vi "PJ1_ui-commu_1_test_4_Harmonics.vi"() -> ()   [LabVIEW 2024]
uses:
  contron/Control 7.ctl
  contron/Control 6.ctl
  contron/Control 5.ctl
  contron/Control 8.ctl
  contol_vr 23/66.ctl
  contol_vr 23/6.ctl
  <vilib>/express/express analysis/Spectral/Block/exnSpectralBlock spectral measurements PSD poly.vi
  <vilib>/express/express analysis/Spectral/XNode/ExpressSpectralMeasurementsBlockNode.xnode
  <vilib>/express/express analysis/Spectral/Block/exnSpectralBlock spectral measurements PSD DDT.vi
panel:
  out "PSD 24-1":dbl
  out "B 24-1":dbl
  in  "Aj 24-1":dbl
  out "B 33-1":dbl
  out "N 33-1":dbl
  in  "Aj 33-1":dbl
  out "B 33-1":dbl
  out "PSD 33-1":dbl
  out "B 33":dbl
  out "N 33":dbl
  in  "Aj 33":dbl
  out "B 33":dbl
  out "PSD 33":dbl
  out "B 33+1":dbl
  out "N 33+1":dbl
  in  "Aj 33+1":dbl
  out "B 33+1":dbl
  out "PSD 33+1":dbl
  out "B24-1":dbl
  out "N 24-1":dbl
  out "B 24":dbl
  out "N 24":dbl
  in  "Aj 24":dbl
  out "B  24":dbl
  out "PSD 24":dbl
  out "B 24+1":dbl
  out "N 24+1":dbl
  in  "Aj 24+1":dbl
  out "B 24+1":dbl
  out "PSD 24+1":dbl
  out "B21-1":dbl
  out "N21-1":dbl
  in  "Aj 21-1":dbl
  out "B  21-1":dbl
  out "PSD 21-1":dbl
  out "B21":dbl
  out "N21":dbl
  in  "Aj 21":dbl
  out "B  21":dbl
  out "PSD 21":dbl
  out "B21+1":dbl
  out "N21+1":dbl
  in  "Aj 21+1":dbl
  out "B  21+1":dbl
  out "PSD 21+1":dbl
  out "B18+1":dbl
  out "N18+1":dbl
  in  "Aj 18+1":dbl
  out "B  18+1":dbl
  out "PSD 18+1":dbl
  out "B18":dbl
  out "N18":dbl
  in  "Aj 18":dbl
  out "B  18":dbl
  out "PSD 18":dbl
  out "B18-1":dbl
  out "N18-1":dbl
  in  "Aj 18-1":dbl
  out "B  18-1":dbl
  out "PSD 18-1":dbl
  out "appended array 2":dbl[](array[numeric])
  out "Array":dbl[](array[numeric])
  in  "start":bool
  out "Clear4":bool
  out "Clear 3":bool
  out "Clear2":bool
  out "check":bool
  out "Clear1":bool
  in  "Baseline":bool
  out "555":bool
  out "6 HZ":bool
  out "7 HZ":bool
  in  "Upper Cut-Off":dbl=40.0
  out "PSD":dynamicdata(graph)
  out "PSD MAX":dbl
  out "Index ที่มากที่สุด":i32
  out "max value":dbl
  out "B 22+1":dbl
  out "N 22+1":dbl
  in  "Aj 22+1":dbl
  out "B 22+1":dbl
  out "PSD 22+1":dbl
  out "B 22":dbl
  out "N 22":dbl
  in  "Aj 22":dbl
  out "B 22":dbl
  out "PSD 22":dbl
  out "B 22-1":dbl
  out "N 22-1":dbl
  in  "Aj 22-1":dbl
  out "B 22-1":dbl
  out "PSD 22-1":dbl
  out "11 Hz":dbl[](array[numeric])
  out "Max Index 11":i32
  out "PSD max 11":dbl
  out "PSD 11+1":dbl
  out "B 11+1":dbl
  in  "Aj 11+1":dbl
  out "N 11+1":dbl
  out "B 11+1":dbl
  out "PSD 11":dbl
  out "B 11":dbl
  in  "Aj 11":dbl
  out "N 11":dbl
  out "B 11":dbl
  out "PSD 11+1":dbl
  out "B 11+1":dbl
  in  "Aj 11+1":dbl
  out "N 11+1":dbl
  out "B 11+1":dbl
  out "8 Hz":dbl[](array[numeric])
  out "Max Index 8":i32
  out "PSD max 8":dbl
  out "B 16+1":dbl
  out "N 16+1":dbl
  in  "Aj  16+1":dbl
  out "B 16+1":dbl
  out "PSD  16+1":dbl
  out "B 16":dbl
  out "N  16":dbl
  in  "Aj  16":dbl
  out "B 16":dbl
  out "PSD  16":dbl
  out "B 16-1":dbl
  out "N  16-1":dbl
  in  "Aj   16-1":dbl
  out "B   16-1":dbl
  out "PSD 16-1":dbl
  out "B 8+1":dbl
  out "N 8+1":dbl
  in  "Aj  8+1":dbl
  out "B  8+1":dbl
  out "PSD 8+1":dbl
  out "B 8":dbl
  out "N  8":dbl
  in  "Aj  8":dbl
  out "B  8":dbl
  out "PSD 8":dbl
  out "B 8-1":dbl
  out "N  8-1":dbl
  in  "Aj  8-1":dbl
  out "B  8-1":dbl
  out "PSD 8-1":dbl
  out "PSD 14+1":dbl
  out "B 14+1":dbl
  in  "Aj 14+1":dbl
  out "N 14+1":dbl
  out "B 14+1":dbl
  out "PSD 14":dbl
  out "B 14":dbl
  in  "Aj 14":dbl
  out "N 14":dbl
  out "B 14":dbl
  out "PSD 14-1":dbl
  out "B 14-1":dbl
  in  "Aj 14-1":dbl
  out "N 14-1":dbl
  out "B 14-1":dbl
  out "PSD7+1":dbl
  out "B7+1":dbl
  in  "Aj7+1":dbl
  out "N7+1":dbl
  out "B7+1":dbl
  out "PSD 7":dbl
  out "B 7":dbl
  in  "Aj 7":dbl
  out "N7":dbl
  out "B7":dbl
  out "7 Hz":dbl[](array[numeric])
  out "Max Index 7":i32
  out "PSD max 7":dbl
  out "PSD 7-1":dbl
  out "B 7-1":dbl
  in  "Aj 7-1":dbl
  out "N7-1":dbl
  out "B7-1":dbl
  out "B12-1":dbl
  out "N12-1":dbl
  in  "Aj 12-1":dbl
  out "B 12-1":dbl
  out "PSD 12-1":dbl
  out "B12":dbl
  out "N12":dbl
  in  "Aj 12":dbl
  out "B12":dbl
  out "PSD 12":dbl
  out "B12+1":dbl
  out "N12+1":dbl
  in  "Aj 12+1":dbl
  out "B 12+1":dbl
  out "PSD 12+1":dbl
  out "B6+1":dbl
  out "N6+1":dbl
  in  "Aj 6+1":dbl
  out "B 6+1":dbl
  out "PSD 6+1":dbl
  out "B6":dbl
  out "N6":dbl
  in  "Aj 6":dbl
  out "B6":dbl
  out "PSD 6":dbl
  out "PSD 6-1":dbl
  out "6 Hz":dbl[](array[numeric])
  out "Max Index 6":i32
  out "PSD max 6":dbl
  out "B 6-1":dbl
  in  "Aj 6-1":dbl
  out "N6-1":dbl
  out "B6-1":dbl
  out "appended array":dbl[][](array[numeric])
  out "Filtered Signal":dynamicdata(graph)
  in  "Lower Cut-Off":dbl=1.0
  out "data":waveform(dbl)(graph) caption="Raw Data"
  in  "number of samples":i32=1000
  in  "rate":dbl=200.0 min=200.0 max=200.0
  out "?":bool
  out "?":bool
  out "?":bool
  out "?":bool
  out "?":bool
  out "?":bool
  out "?":bool
  out "?":bool
  out "?":bool
  out "?":bool
  out "?":bool=TRUE
  out "?":bool=TRUE
  out "?":bool=TRUE
  out "?":bool=TRUE
  out "?":bool=TRUE
  out "?":bool=TRUE
  out "?":bool=TRUE
  out "?":bool=TRUE
  out "?":bool=TRUE
  out "?":bool=TRUE
  out "?":bool
  out "?":bool
  out "?":bool
  out "?":bool
  out "?":bool
  out "?":bool
  out "?":bool
  out "?":bool
  out "?":bool
  out "?":bool
  out "?":bool=TRUE
  out "?":bool=TRUE
  out "?":bool=TRUE
  out "?":bool=TRUE
  out "?":bool=TRUE
  out "?":bool=TRUE
  out "?":bool=TRUE
  out "?":bool=TRUE
  out "?":bool=TRUE
  out "?":bool=TRUE
  out "?":bool
  out "?":bool
  out "?":bool
  out "?":bool
  out "?":bool
  out "?":bool
  out "?":bool
  out "?":bool
  out "?":bool
  out "?":bool
  out "?":bool=TRUE
  out "?":bool=TRUE
  out "?":bool=TRUE
  out "?":bool=TRUE
  out "?":bool=TRUE
  out "?":bool=TRUE
  out "?":bool=TRUE
  out "?":bool=TRUE
  out "?":bool=TRUE
  out "?":bool=TRUE
  out "?":bool
  out "?":bool
  out "?":bool
  out "?":bool
  out "?":bool
  out "?":bool
  out "?":bool
  out "?":bool
  out "?":bool
  out "?":bool
  out "?":bool=TRUE
  out "?":bool=TRUE
  out "?":bool=TRUE
  out "?":bool=TRUE
  out "?":bool=TRUE
  out "?":bool=TRUE
  out "?":bool=TRUE
  out "?":bool=TRUE
  out "?":bool=TRUE
  out "?":bool=TRUE
  out "11 HZ":bool
  out "8 HZ":bool
  in  "Tab Control":enum32{"TAB 1", "TAB 2", "TAB 3", "TAB 4"}(tab)
  out "Emotion 7":bool
  out "Emotion 6":bool
  out "Emotion 5":bool
  out "Emotion 4":bool
  out "ele":T1
  out "Emer":bool
  out "call":T2
  out "commu":T3
  out "Activity":bool
  out "8-2":bool
  out "commu_back":bool
  out "commu_2":bool
  out "commu_1":bool
  out "Emotion":bool
  out "ACC":T4
  out "back_page2":T5
  in  "send":bool
  out "call_back":bool
  out "call_3":bool
  out "call_2":bool
  out "call_1":bool
  out "1 3":bool
  out "1 2":T6
  out "1":bool
  out "String 2":string
  in  "SOS CALLING":bool
  in  "Search Button 2":bool
  out "ele_back":bool
  out "ele_3":bool
  out "ele_2":bool
  out "ele_1":bool
  out "ele_2":bool
  out "ele_3":bool
  out "ele_1":bool
  out "BACK_Page4":bool
  # "6"
  # "7"
  # "8"
  # "11"
  # "MENU"
  # "COMMUNICATION"
  # "SOS CALLING"
  # "Tel."
  # "ELECTRICAL DEVICES"
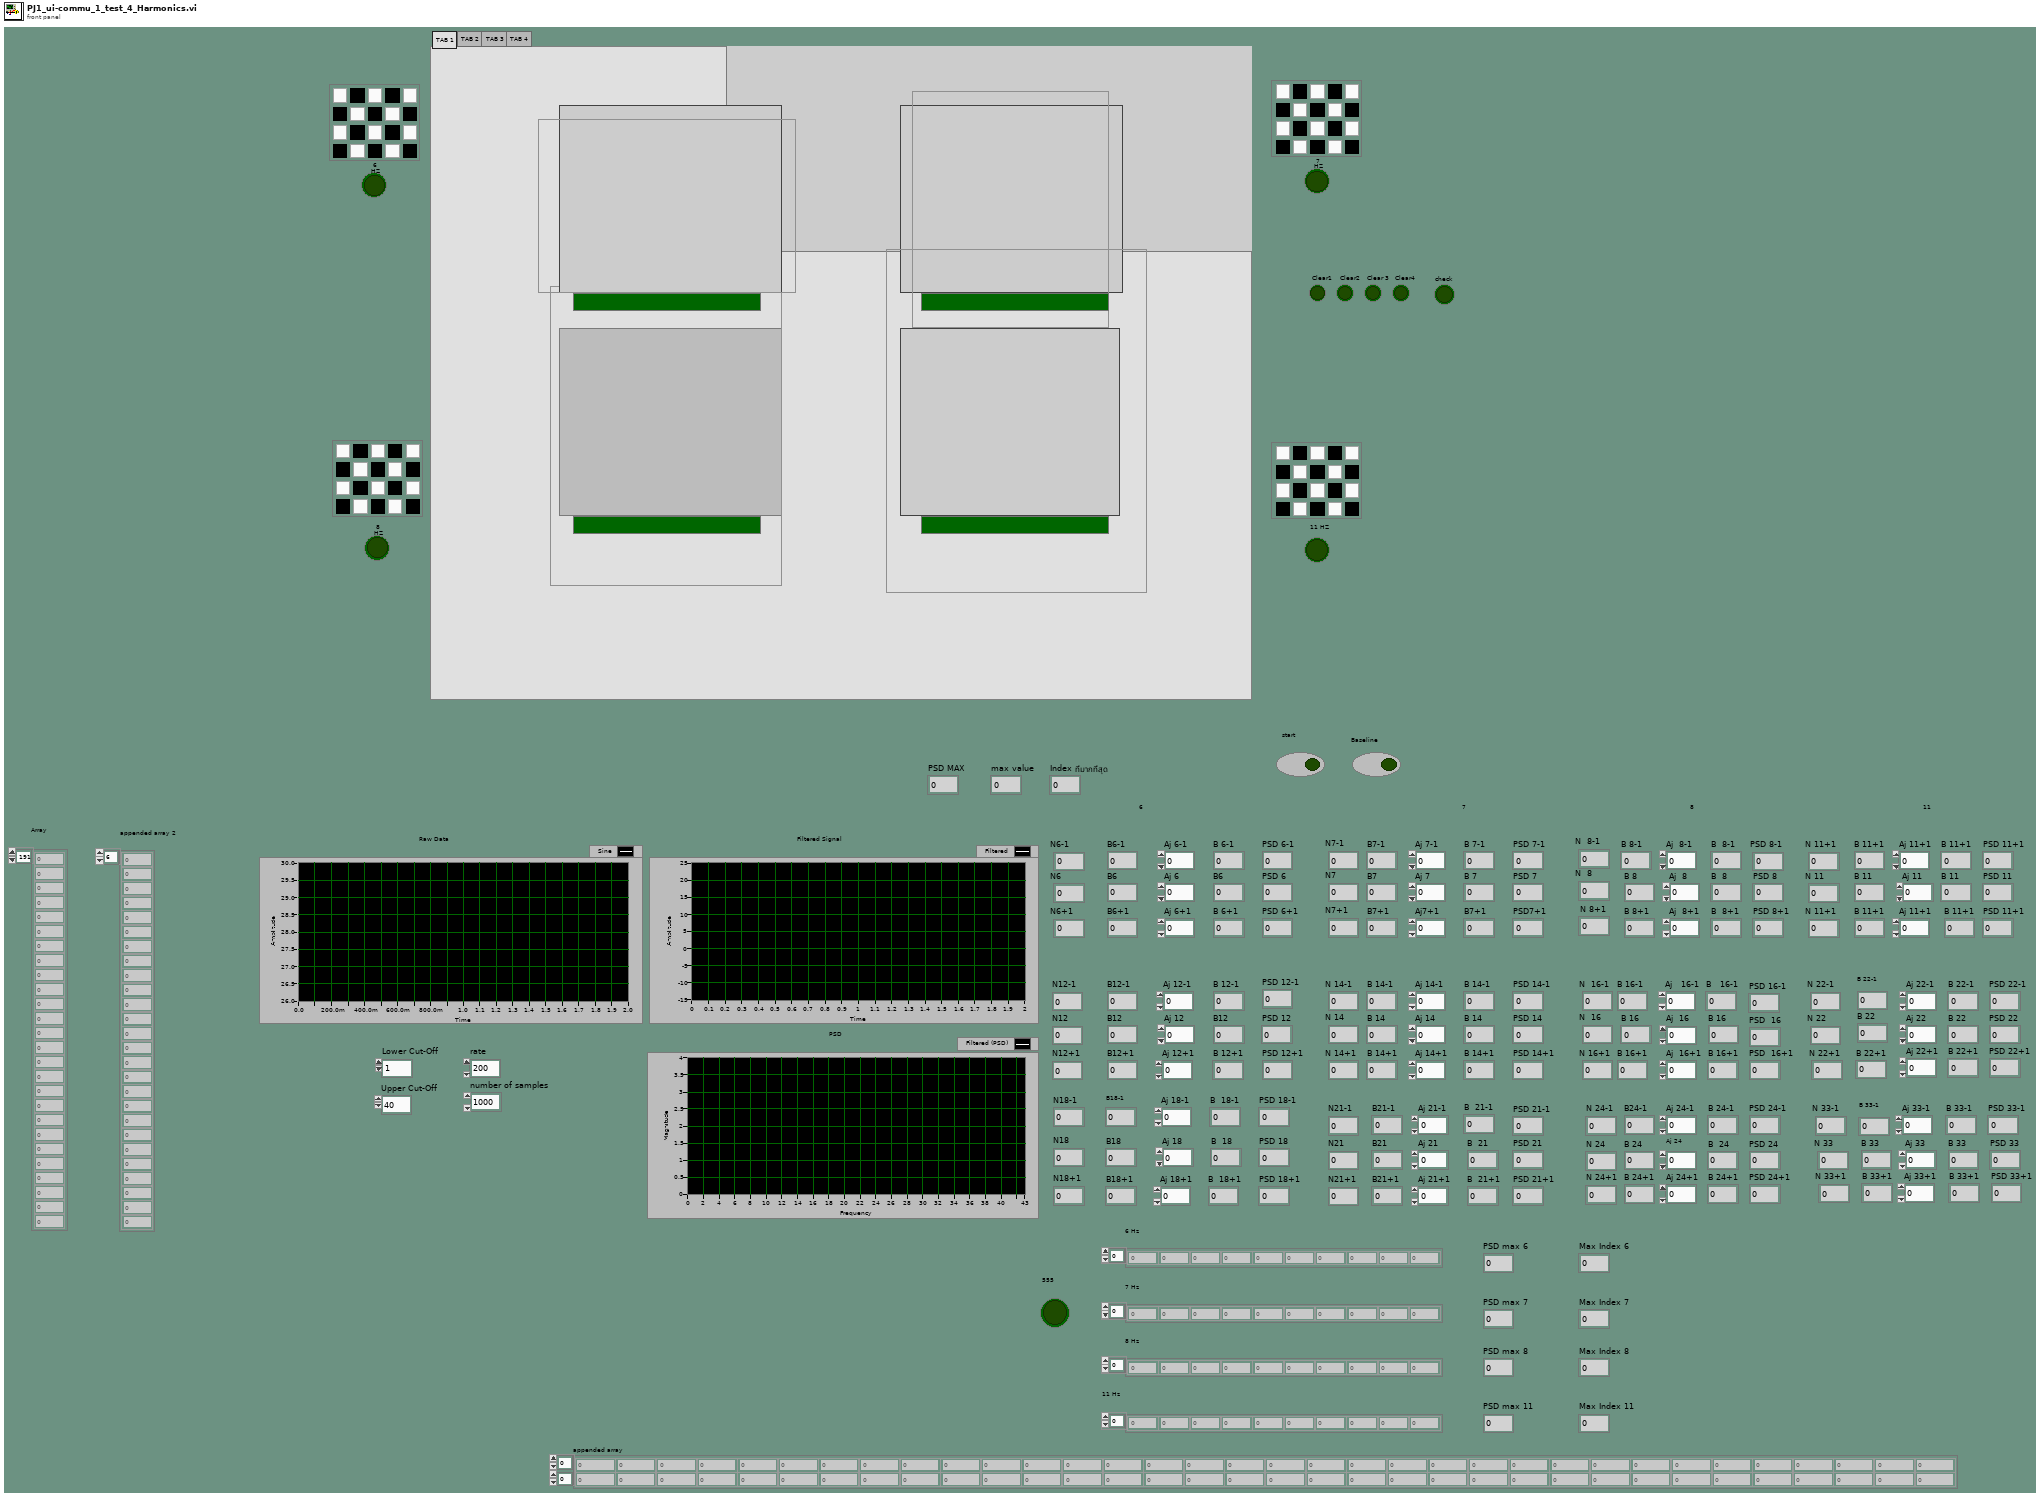
[diagram p1: front panel]
types:
  T1 = typedef "Control 5.ctl" = bool
  T2 = typedef "Control 6.ctl" = bool
  T3 = typedef "Control 7.ctl" = bool
  T4 = typedef "6.ctl" = bool
  T5 = typedef "66.ctl" = bool
  T6 = typedef "Control 8.ctl" = bool
  T7 = cluster{"averaging mode":u16, "weighting mode":u16, "number of averages":u32}
  T8 = cluster{"dB On (F)":bool, "unwrap phase (F)":bool, "convert to degree (F)":bool}
  T9 = enum32{"TAB 1", "TAB 2", "TAB 3", "TAB 4", "TAB 5", "TAB 6", "TAB 7"}
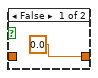
[diagram p2: hidden frame]
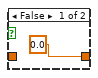
[diagram p4: hidden frame]
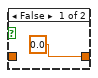
[diagram p6: hidden frame]
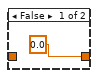
[diagram p8: hidden frame]
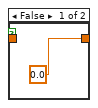
[diagram p10: hidden frame]
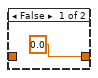
[diagram p12: hidden frame]
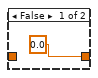
[diagram p14: hidden frame]
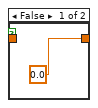
[diagram p16: hidden frame]
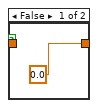
[diagram p18: hidden frame]
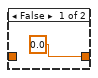
[diagram p20: hidden frame]
diagram:
  n1 = while {
    stop <- FALSE stop-if-true
    n2 = Obtain Queue(name (unnamed)="buffer", element data type=dbl[] []) -> (queue out=w10:refnum<queue>, error out=w9:errorcluster)  [unwired: 3 in, 1 out]
    n3 = Obtain Queue(name (unnamed)="ganglion", element data type=0.0) -> (queue out=w7:refnum<queue>, error out=w8:errorcluster)  [unwired: 3 in, 1 out]
    n4 = while {
      tunnel: w7 -> [w36]
      tunnel: w8 -> [w35]
      shift-right: [w27] -> _
      shift-left: _ -> [_]
      tunnel: w10 -> [w32]
      tunnel: w9 -> [w31]
      tunnel: [w30] -> w13
      tunnel: [w29] -> w12
      stop <- FALSE stop-if-true
      # "เงื่อนไข while"
      n5 = for {
        N: 400 -> [_]
        shift-right: [w38] -> w27
        shift-left: dbl[] [] -> [w40]
        tunnel: [w45] -> _
        tunnel: w35 -> [w46]
        tunnel: [w42] -> _
        tunnel: [w41] -> _
        tunnel: w36 -> [w45]
        # "เคลีย 800 ก่อน"
        # "ตัด 1 วิเเรกออก"
        n6 = Dequeue Element(queue=w45, error in (no error)=w46) -> (queue out=w41:refnum<queue>, element=w39:dbl, error out=w42:errorcluster)  [unwired: 1 in, 1 out]
        n7 = Build Array (concatenate) "Build Array"(w39, w40) -> (w37:dbl[])
        "appended array 2" <- w37
        n8 = Delete From Array "Delete From Array"(array=w37, length=0, index=199 ("index (row)")) -> (array with subset deleted=w38:dbl[])  [unwired: 1 out]
      }
      "Array" <- w27
      n9 = Enqueue Element(queue=w32, element=w27, error in (no error)=w31) -> (queue out=w30:refnum<queue>, error out=w29:errorcluster)  [unwired: 1 in, 1 out]
    }
    n10 = String To IP(1:"127.0.0.1") -> (0:w19:u32)
    n11 = UDP Open(7:w19, 11:u16 5005 ("port")) -> (port=w21:refnum<k16>, 0:w20:errorcluster)  [unwired: 3 in, 1 out]
    n12 = while {
      tunnel: w20 -> [w64]
      tunnel: w21 -> [w62]
      tunnel: [w61] -> w22
      tunnel: [w60] -> w23
      tunnel: [w49] -> w24
      tunnel: w8 -> [w56]
      tunnel: [w55] -> w25
      tunnel: w7 -> [w57]
      stop <- FALSE stop-if-true
      n13 = UDP Read(connection ID=w62, timeout ms (25000)=500, 8:w64) -> (data out=w54:string, error out=w61:errorcluster, 3:w60:refnum<k16>)  [unwired: 1 in, 2 out]
      n14 = Spreadsheet String To Array(delimiter (Tab)=",", format string="%f", spreadsheet string=w54, array type (2D Dbl)=0.0) -> (array=w52:dbl[][])
      n15 = Index Array(array=w52, index (row)=0, index (col)=0 ("disabled index (col)")) -> (element=w47:dbl)
      n16 = Enqueue Element(queue=w57, element=w47, error in (no error)=w56) -> (queue out=w49:refnum<queue>, error out=w55:errorcluster)  [unwired: 1 in, 1 out]
    }
    n17 = UDP Close(connection ID=w23, 8:w22) -> ()  [unwired: 2 out]
    n18 = Release Queue(queue=w24, error in (no error)=w25) -> ()  [unwired: 1 in, 3 out]
    n19 = Release Queue(queue=w13, error in (no error)=w12) -> ()  [unwired: 1 in, 3 out]
    n20 = while {
      tunnel: w10 -> [w246]
      tunnel: w9 -> [w245]
      stop <- FALSE stop-if-true
      n21 = Dequeue Element(queue=w246, error in (no error)=w245) -> (element=w243:dbl[])  [unwired: 1 in, 3 out]
      n22 = Bundle By Name("dt"=0.005, "Y"=w243) -> (w242:waveform(dbl))  [unwired: 1 in]
      "data" <- w242
      n23 = Divide(x="number of samples", y="rate") -> (x/y=w109:dbl)
      n24 = Divide(x=33.0, y=w109) -> (x/y=w72:dbl)
      n25 = Divide(x=11.0, y=w109) -> (x/y=w354:dbl)
      n26 = Divide(x=22.0, y=w109) -> (x/y=w312:dbl)
      n27 = Divide(x=16.0, y=w109) -> (x/y=w388:dbl)
      n28 = call "Filter"("Lower Cut-Off"="Lower Cut-Off", "Upper Cut-Off"="Upper Cut-Off", "Signal"=w242) -> ("Filtered Signal"=w253:dynamicdata)  [unwired: 7 in, 1 out]
      "Filtered Signal" <- w253
      n29 = Divide(x=21.0, y=w109) -> (x/y=w160:dbl)
      n30 = Divide(x=14.0, y=w109) -> (x/y=w459:dbl)
      n31 = Divide(x=24.0, y=w109) -> (x/y=w115:dbl)
      n32 = Divide(x=8.0, y=w109) -> (x/y=w116:dbl)
      n33 = Divide(x=7.0, y=w109) -> (x/y=w476:dbl)
      n34 = Decrement(x=w354) -> (x-1=w385:dbl)
      n35 = Increment(x=w354) -> (x+1=w353:dbl)
      n36 = Decrement(x=w72) -> (x-1=w75:dbl)
      n37 = Increment(x=w72) -> (x+1=w69:dbl)
      n38 = Increment(x=w312) -> (x+1=w302:dbl)
      n39 = Decrement(x=w312) -> (x-1=w326:dbl)
      n40 = Increment(x=w115) -> (x+1=w114:dbl)
      n41 = Decrement(x=w115) -> (x-1=w119:dbl)
      n42 = Increment(x=w116) -> (x+1=w426:dbl)
      n43 = Decrement(x=w388) -> (x-1=w411:dbl)
      n44 = Decrement(x=w116) -> (x-1=w448:dbl)
      n45 = Increment(x=w388) -> (x+1=w387:dbl)
      n46 = xnode "Spectral Measurements"("Signals"=w253) -> ("PSD"=w279:dynamicdata)  [unwired: 1 in, 1 out]
      "PSD" <- w279
      n47 = Decrement(x=w476) -> (x-1=w517:dbl)
      "PSD 7-1" <- w517
      n48 = Decrement(x=w459) -> (x-1=w488:dbl)
      n49 = Increment(x=w476) -> (x+1=w502:dbl)
      n50 = Increment(x=w459) -> (x+1=w465:dbl)
      n51 = Divide(x=18.0, y=w109) -> (x/y=w205:dbl)
      n52 = Increment(x=w160) -> (x+1=w159:dbl)
      n53 = Divide(x=12.0, y=w109) -> (x/y=w545:dbl)
      n54 = Divide(x=6.0, y=w109) -> (x/y=w594:dbl)
      n55 = Decrement(x=w160) -> (x-1=w162:dbl)
      n56 = Decrement(x=w594) -> (x-1=w607:dbl)
      n57 = Increment(x=w594) -> (x+1=w583:dbl)
      n58 = Decrement(x=w205) -> (x-1=w240:dbl)
      n59 = call "Convert from Dynamic Data"("Dynamic Data Type"=w279) -> ("Array"=w622:dbl[])  [unwired: 3 in]
      n60 = Decrement(x=w545) -> (x-1=w550:dbl)
      n61 = Increment(x=w205) -> (x+1=w204:dbl)
      n62 = Increment(x=w545) -> (x+1=w544:dbl)
      n63 = feedback #1() -> (w107:dbl)  [unwired: 1 in]
      "B 33" <- w107
      n64 = feedback #2() -> (w106:dbl)  [unwired: 1 in]
      "B 33-1" <- w106
      n65 = feedback #3() -> (w108:dbl)  [unwired: 1 in]
      "B 33+1" <- w108
      n66 = Build Array(w622) -> (w73:dbl[][])
      "appended array" <- w73
      n67 = Index Array(array=w73, index (row)=0, index (col)=w69) -> (element=w105:dbl)
      "PSD 33+1" <- w105
      n68 = Index Array(array=w73, index (row)=0 ("disabled index (row)"), index (col)=w72) -> (element=w95:dbl)
      "PSD 33" <- w95
      n69 = Index Array(array=w73, index (row)=0 ("disabled index (row)"), index (col)=w75) -> (element=w85:dbl)
      "PSD 33-1" <- w85
      n70 = Index Array(array=w73, index (row)=0 ("disabled index (row)"), index (col)=w326) -> (element=w324:dbl)
      "PSD 22-1" <- w324
      n71 = Index Array(array=w73, index (row)=0 ("disabled index (row)"), index (col)=w302) -> (element=w300:dbl)
      "PSD 22+1" <- w300
      n72 = Index Array(array=w73, index (row)=0, index (col)=w353) -> (element=w342:dbl)
      "PSD 11+1" <- w342
      n73 = Index Array(array=w73, index (row)=0 ("disabled index (row)"), index (col)=w312) -> (element=w313:dbl)
      "PSD 22" <- w313
      n74 = Index Array(array=w73, index (row)=0, index (col)=w354) -> (element=w355:dbl)
      "PSD 11" <- w355
      n75 = Index Array(array=w73, index (row)=0, index (col)=w385) -> (element=w366:dbl)
      "PSD 11+1" <- w366
      n76 = Index Array(array=w73, index (row)=0, index (col)=w411) -> (element=w422:dbl)
      "PSD 16-1" <- w422
      n77 = Index Array(array=w73, index (row)=0 ("disabled index (row)"), index (col)=w387) -> (element=w399:dbl)
      "PSD  16+1" <- w399
      n78 = Index Array(array=w73, index (row)=0 ("disabled index (row)"), index (col)=w388) -> (element=w401:dbl)
      "PSD  16" <- w401
      n79 = case shown="False" "Baseline" {
        tunnel: w95 -> [_ w631]
        tunnel: [w630 w631] -> w94
        tunnel: w107 -> [w630 _]
        frame False {
        }
        frame True {
        }
      }
      n80 = case shown="False" "Baseline" {
        tunnel: w85 -> [_ w635]
        tunnel: [w634 w635] -> w76
        tunnel: w106 -> [w634 _]
        frame False {
        }
        frame True {
        }
      }
      n81 = Index Array(array=w73, index (row)=0, index (col)=w426) -> (element=w424:dbl)
      "PSD 8+1" <- w424
      n82 = case shown="False" "Baseline" {
        tunnel: w105 -> [_ w627]
        tunnel: [w626 w627] -> w96
        tunnel: w108 -> [w626 _]
        frame False {
        }
        frame True {
        }
      }
      n83 = Index Array(array=w73, index (row)=0, index (col)=w116) -> (element=w446:dbl)
      "PSD 8" <- w446
      n84 = Index Array(array=w73, index (row)=0, index (col)=w448) -> (element=w447:dbl)
      "PSD 8-1" <- w447
      n85 = Index Array(array=w73, index (row)=0 ("disabled index (row)"), index (col)=w114) -> (element=w121:dbl)
      "PSD 24+1" <- w121
      n86 = Index Array(array=w73, index (row)=0 ("disabled index (row)"), index (col)=w115) -> (element=w133:dbl)
      "PSD 24" <- w133
      n87 = Index Array(array=w73, index (row)=0 ("disabled index (row)"), index (col)=w119) -> (element=w145:dbl)
      "PSD 24-1" <- w145
      n88 = Index Array(array=w73, index (row)=0, index (col)=w465) -> (element=w466:dbl)
      "PSD 14+1" <- w466
      n89 = Index Array(array=w73, index (row)=0, index (col)=w488) -> (element=w490:dbl)
      "PSD 14-1" <- w490
      n90 = Index Array(array=w73, index (row)=0, index (col)=w517) -> ()  [unwired: 1 out]
      n91 = Index Array(array=w73, index (row)=0 ("disabled index (row)"), index (col)=w476) -> (element=w514:dbl)
      "PSD 7" <- w514
      n92 = Index Array(array=w73, index (row)=0, index (col)=w459) -> (element=w477:dbl)
      "PSD 14" <- w477
      n93 = Index Array(array=w73, index (row)=0, index (col)=w502) -> (element=w503:dbl)
      "PSD7+1" <- w503
      n94 = Index Array(array=w73, index (row)=0 ("disabled index (row)"), index (col)=w159) -> (element=w163:dbl)
      "PSD 21+1" <- w163
      n95 = Index Array(array=w73, index (row)=0 ("disabled index (row)"), index (col)=w160) -> (element=w175:dbl)
      "PSD 21" <- w175
      n96 = feedback-in #1(w94) -> ()
      n97 = feedback-in #2(w76) -> ()
      n98 = feedback-in #3(w96) -> ()
      n99 = feedback #4() -> (w255:dbl)  [unwired: 1 in]
      "B 22" <- w255
      n100 = case shown="False" "Baseline" {
        tunnel: w313 -> [_ w681]
        tunnel: [w680 w681] -> w315
        tunnel: w255 -> [w680 _]
        frame False {
        }
        frame True {
        }
      }
      n101 = feedback-in #4(w315) -> ()
      n102 = Index Array(array=w73, index (row)=0 ("disabled index (row)"), index (col)=w162) -> (element=w187:dbl)
      "PSD 21-1" <- w187
      n103 = feedback #5() -> (w256:dbl)  [unwired: 1 in]
      "B 22-1" <- w256
      n104 = case shown="False" "Baseline" {
        tunnel: w324 -> [_ w685]
        tunnel: [w684 w685] -> w335
        tunnel: w256 -> [w684 _]
        frame False {
        }
        frame True {
        }
      }
      n105 = feedback-in #5(w335) -> ()
      n106 = feedback #6() -> (w254:dbl)  [unwired: 1 in]
      "B 22+1" <- w254
      n107 = case shown="False" "Baseline" {
        tunnel: w300 -> [_ w677]
        tunnel: [w676 w677] -> w311
        tunnel: w254 -> [w676 _]
        frame False {
        }
        frame True {
        }
      }
      n108 = feedback-in #6(w311) -> ()
      n109 = feedback #7() -> (w258:dbl)  [unwired: 1 in]
      "B 11" <- w258
      n110 = case shown="False" "Baseline" {
        tunnel: w355 -> [_ w693]
        tunnel: [w692 w693] -> w356
        tunnel: w258 -> [w692 _]
        frame False {
        }
        frame True {
        }
      }
      n111 = feedback-in #7(w356) -> ()
      n112 = feedback #8() -> (w259:dbl)  [unwired: 1 in]
      "B 11+1" <- w259
      n113 = case shown="True" "Baseline" {
        tunnel: w366 -> [_ w697]
        tunnel: [w696 w697] -> w367
        tunnel: w259 -> [w696 _]
        frame False {
        }
        frame True {
        }
      }
      n114 = feedback-in #8(w367) -> ()
      n115 = feedback #9() -> (w257:dbl)  [unwired: 1 in]
      "B 11+1" <- w257
      n116 = case shown="False" "Baseline" {
        tunnel: w342 -> [_ w689]
        tunnel: [w688 w689] -> w343
        tunnel: w257 -> [w688 _]
        frame False {
        }
        frame True {
        }
      }
      n117 = feedback-in #9(w343) -> ()
      n118 = feedback #10() -> (w132:dbl)  [unwired: 1 in]
      "B 24+1" <- w132
      n119 = case shown="True" "Baseline" {
        tunnel: w121 -> [_ w639]
        tunnel: [w638 w639] -> w124
        tunnel: w132 -> [w638 _]
        frame False {
        }
        frame True {
        }
      }
      n120 = feedback-in #10(w124) -> ()
      n121 = Add(x=w107, y="Aj 33") -> (x+y=w90:dbl)
      "B 33" <- w90
      n122 = Index Array(array=w73, index (row)=0 ("disabled index (row)"), index (col)=w204) -> (element=w202:dbl)
      "PSD 18+1" <- w202
      n123 = Index Array(array=w73, index (row)=0 ("disabled index (row)"), index (col)=w205) -> (element=w216:dbl)
      "PSD 18" <- w216
      n124 = Add(x=w106, y="Aj 33-1") -> (x+y=w80:dbl)
      "B 33-1" <- w80
      n125 = Add(x=w108, y="Aj 33+1") -> (x+y=w100:dbl)
      "B 33+1" <- w100
      n126 = feedback #11() -> (w262:dbl)  [unwired: 1 in]
      "B 16-1" <- w262
      n127 = case shown="True" "Baseline" {
        tunnel: w422 -> [_ w709]
        tunnel: [w708 w709] -> w412
        tunnel: w262 -> [w708 _]
        frame False {
        }
        frame True {
        }
      }
      n128 = feedback-in #11(w412) -> ()
      n129 = feedback #12() -> (w260:dbl)  [unwired: 1 in]
      "B 16+1" <- w260
      n130 = case shown="True" "Baseline" {
        tunnel: w399 -> [_ w701]
        tunnel: [w700 w701] -> w390
        tunnel: w260 -> [w700 _]
        frame False {
        }
        frame True {
        }
      }
      n131 = feedback-in #12(w390) -> ()
      n132 = feedback #13() -> (w261:dbl)  [unwired: 1 in]
      "B 16" <- w261
      n133 = case shown="True" "Baseline" {
        tunnel: w401 -> [_ w705]
        tunnel: [w704 w705] -> w410
        tunnel: w261 -> [w704 _]
        frame False {
        }
        frame True {
        }
      }
      n134 = feedback-in #13(w410) -> ()
      n135 = feedback #14() -> (w263:dbl)  [unwired: 1 in]
      "B 8+1" <- w263
      n136 = case shown="True" "Baseline" {
        tunnel: w424 -> [_ w713]
        tunnel: [w712 w713] -> w435
        tunnel: w263 -> [w712 _]
        frame False {
        }
        frame True {
        }
      }
      n137 = feedback-in #14(w435) -> ()
      n138 = Add(x=w255, y="Aj 22") -> (x+y=w319:dbl)
      "B 22" <- w319
      n139 = feedback #15() -> (w264:dbl)  [unwired: 1 in]
      "B 8" <- w264
      n140 = case shown="True" "Baseline" {
        tunnel: w446 -> [_ w717]
        tunnel: [w716 w717] -> w437
        tunnel: w264 -> [w716 _]
        frame False {
        }
        frame True {
        }
      }
      n141 = feedback-in #15(w437) -> ()
      n142 = Add(x=w256, y="Aj 22-1") -> (x+y=w331:dbl)
      "B 22-1" <- w331
      n143 = Index Array(array=w73, index (row)=0 ("disabled index (row)"), index (col)=w240) -> (element=w229:dbl)
      "PSD 18-1" <- w229
      n144 = Add(x=w254, y="Aj 22+1") -> (x+y=w307:dbl)
      "B 22+1" <- w307
      n145 = feedback #16() -> (w265:dbl)  [unwired: 1 in]
      "B 8-1" <- w265
      n146 = case shown="True" "Baseline" {
        tunnel: w447 -> [_ w721]
        tunnel: [w720 w721] -> w458
        tunnel: w265 -> [w720 _]
        frame False {
        }
        frame True {
        }
      }
      n147 = feedback-in #16(w458) -> ()
      n148 = Multiply(x=w107, y=4.0) -> (x*y=w87:dbl)
      "N 33" <- w87
      n149 = Index Array(array=w73, index (row)=0 ("disabled index (row)"), index (col)=w583) -> (element=w581:dbl)
      "PSD 6+1" <- w581
      n150 = Index Array(array=w73, index (row)=0, index (col)=w550) -> (element=w549:dbl)
      "PSD 12-1" <- w549
      n151 = Index Array(array=w73, index (row)=0 ("disabled index (row)"), index (col)=w545) -> (element=w546:dbl)
      "PSD 12" <- w546
      n152 = Index Array(array=w73, index (row)=0 ("disabled index (row)"), index (col)=w544) -> (element=w542:dbl)
      "PSD 12+1" <- w542
      n153 = Multiply(x=w106, y=4.0) -> (x*y=w83:dbl)
      "N 33-1" <- w83
      n154 = Index Array(array=w73, index (row)=0, index (col)=w594) -> (element=w595:dbl)
      "PSD 6" <- w595
      n155 = Index Array(array=w73, index (row)=0, index (col)=w607) -> (element=w614:dbl)
      "PSD 6-1" <- w614
      n156 = feedback #17() -> (w134:dbl)  [unwired: 1 in]
      "B 24" <- w134
      n157 = case shown="True" "Baseline" {
        tunnel: w133 -> [_ w643]
        tunnel: [w642 w643] -> w142
        tunnel: w134 -> [w642 _]
        frame False {
        }
        frame True {
        }
      }
      n158 = feedback-in #17(w142) -> ()
      n159 = Multiply(x=w108, y=4.0) -> (x*y=w103:dbl)
      "N 33+1" <- w103
      n160 = Add(x=w258, y="Aj 11") -> (x+y=w360:dbl)
      "B 11" <- w360
      n161 = feedback #18() -> (w266:dbl)  [unwired: 1 in]
      "B 14+1" <- w266
      n162 = case shown="True" "Baseline" {
        tunnel: w466 -> [_ w725]
        tunnel: [w724 w725] -> w467
        tunnel: w266 -> [w724 _]
        frame False {
        }
        frame True {
        }
      }
      n163 = feedback-in #18(w467) -> ()
      n164 = Add(x=w259, y="Aj 11+1") -> (x+y=w371:dbl)
      "B 11+1" <- w371
      n165 = Add(x=w257, y="Aj 11+1") -> (x+y=w347:dbl)
      "B 11+1" <- w347
      n166 = Multiply(x=w255, y=4.0) -> (x*y=w322:dbl)
      "N 22" <- w322
      n167 = Multiply(x=w256, y=4.0) -> (x*y=w328:dbl)
      "N 22-1" <- w328
      n168 = Multiply(x=w254, y=4.0) -> (x*y=w304:dbl)
      "N 22+1" <- w304
      n169 = feedback #19() -> (w268:dbl)  [unwired: 1 in]
      "B 14-1" <- w268
      n170 = case shown="True" "Baseline" {
        tunnel: w490 -> [_ w733]
        tunnel: [w732 w733] -> w491
        tunnel: w268 -> [w732 _]
        frame False {
        }
        frame True {
        }
      }
      n171 = feedback-in #19(w491) -> ()
      n172 = feedback #20() -> (w174:dbl)  [unwired: 1 in]
      "B21+1" <- w174
      n173 = case shown="True" "Baseline" {
        tunnel: w163 -> [_ w651]
        tunnel: [w650 w651] -> w166
        tunnel: w174 -> [w650 _]
        frame False {
        }
        frame True {
        }
      }
      n174 = feedback-in #20(w166) -> ()
      n175 = feedback #21() -> (w154:dbl)  [unwired: 1 in]
      "B24-1" <- w154
      n176 = case shown="True" "Baseline" {
        tunnel: w145 -> [_ w647]
        tunnel: [w646 w647] -> w146
        tunnel: w154 -> [w646 _]
        frame False {
        }
        frame True {
        }
      }
      n177 = feedback-in #21(w146) -> ()
      n178 = Greater?(x=w95, y=w90) -> (0:w89:bool)
      n179 = Add(x=w262, y="Aj   16-1") -> (x+y=w416:dbl)
      "B   16-1" <- w416
      n180 = Greater?(x=w85, y=w80) -> (0:w81:bool)
      n181 = Multiply(x=w258, y=4.0) -> (x*y=w363:dbl)
      "N 11" <- w363
      n182 = Greater?(x=w105, y=w100) -> (0:w101:bool)
      n183 = Add(x=w261, y="Aj  16") -> (x+y=w406:dbl)
      "B 16" <- w406
      n184 = Add(x=w263, y="Aj  8+1") -> (x+y=w431:dbl)
      "B  8+1" <- w431
      n185 = Less?(x=w95, y=w87) -> (x < y?=w88:bool)
      n186 = feedback #22() -> (w267:dbl)  [unwired: 1 in]
      "B 14" <- w267
      n187 = case shown="True" "Baseline" {
        tunnel: w477 -> [_ w729]
        tunnel: [w728 w729] -> w479
        tunnel: w267 -> [w728 _]
        frame False {
        }
        frame True {
        }
      }
      n188 = feedback-in #22(w479) -> ()
      n189 = Less?(x=w85, y=w83) -> (x < y?=w82:bool)
      n190 = Multiply(x=w259, y=4.0) -> (x*y=w374:dbl)
      "N 11+1" <- w374
      n191 = Less?(x=w105, y=w103) -> (x < y?=w102:bool)
      n192 = Add(x=w264, y="Aj  8") -> (x+y=w441:dbl)
      "B  8" <- w441
      n193 = Multiply(x=w257, y=4.0) -> (x*y=w350:dbl)
      "N 11+1" <- w350
      n194 = Add(x=w265, y="Aj  8-1") -> (x+y=w454:dbl)
      "B  8-1" <- w454
      n195 = Greater?(x=w313, y=w319) -> (0:w320:bool)
      n196 = Greater?(x=w324, y=w331) -> (0:w330:bool)
      n197 = feedback #23() -> (w176:dbl)  [unwired: 1 in]
      "B21" <- w176
      n198 = case shown="False" "Baseline" {
        tunnel: w175 -> [_ w655]
        tunnel: [w654 w655] -> w184
        tunnel: w176 -> [w654 _]
        frame False {
        }
        frame True {
        }
      }
      n199 = feedback-in #23(w184) -> ()
      n200 = Add(x=w260, y="Aj  16+1") -> (x+y=w394:dbl)
      "B 16+1" <- w394
      n201 = Greater?(x=w300, y=w307) -> (0:w306:bool)
      n202 = Less?(x=w313, y=w322) -> (x < y?=w321:bool)
      n203 = Less?(x=w324, y=w328) -> (x < y?=w329:bool)
      n204 = Less?(x=w300, y=w304) -> (x < y?=w305:bool)
      n205 = Multiply(x=w262, y=4.0) -> (x*y=w419:dbl)
      "N  16-1" <- w419
      n206 = Add(x=w266, y="Aj 14+1") -> (x+y=w471:dbl)
      "B 14+1" <- w471
      n207 = Multiply(x=w260, y=4.0) -> (x*y=w397:dbl)
      "N 16+1" <- w397
      n208 = Multiply(x=w261, y=4.0) -> (x*y=w403:dbl)
      "N  16" <- w403
      n209 = Multiply(x=w263, y=4.0) -> (x*y=w428:dbl)
      "N 8+1" <- w428
      n210 = Multiply(x=w264, y=4.0) -> (x*y=w444:dbl)
      "N  8" <- w444
      n211 = Greater?(x=w355, y=w360) -> (0:w361:bool)
      n212 = feedback #24() -> (w270:dbl)  [unwired: 1 in]
      "B7" <- w270
      n213 = case shown="True" "Baseline" {
        tunnel: w514 -> [_ w741]
        tunnel: [w740 w741] -> w518
        tunnel: w270 -> [w740 _]
        frame False {
        }
        frame True {
        }
      }
      n214 = feedback-in #24(w518) -> ()
      n215 = Add(x=w268, y="Aj 14-1") -> (x+y=w495:dbl)
      "B 14-1" <- w495
      n216 = And(x=w88, y=w89) -> (x .and. y?=w91:bool)
      n217 = Subtract(x=w95, y=w90) -> (x-y=w92:dbl)
      n218 = Multiply(x=w265, y=4.0) -> (x*y=w451:dbl)
      "N  8-1" <- w451
      n219 = And(x=w82, y=w81) -> (x .and. y?=w79:bool)
      n220 = Less?(x=w355, y=w363) -> (x < y?=w362:bool)
      n221 = Subtract(x=w85, y=w80) -> (x-y=w78:dbl)
      n222 = Greater?(x=w366, y=w371) -> (0:w372:bool)
      n223 = And(x=w102, y=w101) -> (x .and. y?=w99:bool)
      n224 = Add(x=w132, y="Aj 24+1") -> (x+y=w123:dbl)
      "B 24+1" <- w123
      n225 = Subtract(x=w105, y=w100) -> (x-y=w98:dbl)
      n226 = Add(x=w134, y="Aj 24") -> (x+y=w143:dbl)
      "B  24" <- w143
      n227 = feedback #25() -> (w215:dbl)  [unwired: 1 in]
      "B18+1" <- w215
      n228 = case shown="True" "Baseline" {
        tunnel: w202 -> [_ w663]
        tunnel: [w662 w663] -> w207
        tunnel: w215 -> [w662 _]
        frame False {
        }
        frame True {
        }
      }
      n229 = feedback-in #25(w207) -> ()
      n230 = feedback #26() -> (w271:dbl)  [unwired: 1 in]
      "B7-1" <- w271
      n231 = case shown="True" "Baseline" {
        tunnel: w517 -> [_ w745]
        tunnel: [w744 w745] -> w531
        tunnel: w271 -> [w744 _]
        frame False {
        }
        frame True {
        }
      }
      n232 = feedback-in #26(w531) -> ()
      n233 = Less?(x=w366, y=w374) -> (x < y?=w373:bool)
      n234 = Greater?(x=w342, y=w347) -> (0:w348:bool)
      n235 = Add(x=w154, y="Aj 24-1") -> (x+y=w144:dbl)
      "B 24-1" <- w144
      n236 = Less?(x=w342, y=w350) -> (x < y?=w349:bool)
      n237 = feedback #27() -> (w196:dbl)  [unwired: 1 in]
      "B21-1" <- w196
      n238 = case shown="True" "Baseline" {
        tunnel: w187 -> [_ w659]
        tunnel: [w658 w659] -> w188
        tunnel: w196 -> [w658 _]
        frame False {
        }
        frame True {
        }
      }
      n239 = feedback-in #27(w188) -> ()
      n240 = Add(x=w267, y="Aj 14") -> (x+y=w483:dbl)
      "B 14" <- w483
      n241 = Multiply(x=w266, y=4.0) -> (x*y=w474:dbl)
      "N 14+1" <- w474
      n242 = Multiply(x=w132, y=4.0) -> (x*y=w130:dbl)
      "N 24+1" <- w130
      n243 = feedback #28() -> (w269:dbl)  [unwired: 1 in]
      n244 = case shown="True" "Baseline" {
        tunnel: w503 -> [_ w737]
        tunnel: [w736 w737] -> w505
        tunnel: w269 -> [w736 _]
        frame False {
        }
        frame True {
        }
      }
      n245 = feedback-in #28(w505) -> ()
      n246 = And(x=w321, y=w320) -> (x .and. y?=w318:bool)
      n247 = Subtract(x=w313, y=w319) -> (x-y=w317:dbl)
      n248 = And(x=w329, y=w330) -> (x .and. y?=w332:bool)
      n249 = Subtract(x=w324, y=w331) -> (x-y=w333:dbl)
      n250 = And(x=w305, y=w306) -> (x .and. y?=w308:bool)
      n251 = Greater?(x=w422, y=w416) -> (0:w417:bool)
      n252 = Subtract(x=w300, y=w307) -> (x-y=w309:dbl)
      n253 = Greater?(x=w399, y=w394) -> (0:w395:bool)
      n254 = Multiply(x=w134, y=4.0) -> (x*y=w136:dbl)
      "N 24" <- w136
      n255 = Greater?(x=w401, y=w406) -> (0:w405:bool)
      n256 = Multiply(x=w268, y=4.0) -> (x*y=w498:dbl)
      "N 14-1" <- w498
      n257 = Greater?(x=w424, y=w431) -> (0:w430:bool)
      n258 = Less?(x=w422, y=w419) -> (x < y?=w418:bool)
      n259 = Less?(x=w399, y=w397) -> (x < y?=w396:bool)
      n260 = feedback #29() -> (w274:dbl)  [unwired: 1 in]
      "B12-1" <- w274
      n261 = case shown="True" "Baseline" {
        tunnel: w549 -> [_ w757]
        tunnel: [w756 w757] -> w561
        tunnel: w274 -> [w756 _]
        frame False {
        }
        frame True {
        }
      }
      n262 = feedback-in #29(w561) -> ()
      n263 = Less?(x=w401, y=w403) -> (x < y?=w404:bool)
      n264 = Less?(x=w424, y=w428) -> (x < y?=w429:bool)
      n265 = Greater?(x=w446, y=w441) -> (0:w442:bool)
      n266 = feedback #30() -> (w275:dbl)  [unwired: 1 in]
      "B6+1" <- w275
      n267 = case shown="True" "Baseline" {
        tunnel: w581 -> [_ w761]
        tunnel: [w760 w761] -> w584
        tunnel: w275 -> [w760 _]
        frame False {
        }
        frame True {
        }
      }
      n268 = feedback-in #30(w584) -> ()
      n269 = Multiply(x=w154, y=4.0) -> (x*y=w152:dbl)
      "N 24-1" <- w152
      n270 = feedback #31() -> (w218:dbl)  [unwired: 1 in]
      "B18" <- w218
      n271 = case shown="True" "Baseline" {
        tunnel: w216 -> [_ w667]
        tunnel: [w666 w667] -> w226
        tunnel: w218 -> [w666 _]
        frame False {
        }
        frame True {
        }
      }
      n272 = feedback-in #31(w226) -> ()
      n273 = Greater?(x=w447, y=w454) -> (0:w453:bool)
      n274 = Less?(x=w446, y=w444) -> (x < y?=w443:bool)
      n275 = And(x=w362, y=w361) -> (x .and. y?=w359:bool)
      n276 = Subtract(x=w355, y=w360) -> (x-y=w358:dbl)
      n277 = Less?(x=w447, y=w451) -> (x < y?=w452:bool)
      n278 = feedback #32() -> (w272:dbl)  [unwired: 1 in]
      "B12+1" <- w272
      n279 = case shown="True" "Baseline" {
        tunnel: w542 -> [_ w749]
        tunnel: [w748 w749] -> w579
        tunnel: w272 -> [w748 _]
        frame False {
        }
        frame True {
        }
      }
      n280 = feedback-in #32(w579) -> ()
      n281 = And(x=w373, y=w372) -> (x .and. y?=w370:bool)
      n282 = Subtract(x=w366, y=w371) -> (x-y=w369:dbl)
      n283 = Multiply(x=w267, y=4.0) -> (x*y=w486:dbl)
      "N 14" <- w486
      n284 = feedback #33() -> (w276:dbl)  [unwired: 1 in]
      "B6" <- w276
      n285 = case shown="True" "Baseline" {
        tunnel: w595 -> [_ w765]
        tunnel: [w764 w765] -> w605
        tunnel: w276 -> [w764 _]
        frame False {
        }
        frame True {
        }
      }
      n286 = feedback-in #33(w605) -> ()
      n287 = feedback #34() -> (w277:dbl)  [unwired: 1 in]
      "B6-1" <- w277
      n288 = case shown="True" "Baseline" {
        tunnel: w614 -> [_ w769]
        tunnel: [w768 w769] -> w606
        tunnel: w277 -> [w768 _]
        frame False {
        }
        frame True {
        }
      }
      n289 = feedback-in #34(w606) -> ()
      n290 = And(x=w349, y=w348) -> (x .and. y?=w346:bool)
      n291 = Subtract(x=w342, y=w347) -> (x-y=w345:dbl)
      n292 = feedback #35() -> (w273:dbl)  [unwired: 1 in]
      "B12" <- w273
      n293 = case shown="True" "Baseline" {
        tunnel: w546 -> [_ w753]
        tunnel: [w752 w753] -> w562
        tunnel: w273 -> [w752 _]
        frame False {
        }
        frame True {
        }
      }
      n294 = feedback-in #35(w562) -> ()
      n295 = Greater?(x=w466, y=w471) -> (0:w472:bool)
      n296 = Add(x=w270, y="Aj 7") -> (x+y=w522:dbl)
      "B 7" <- w522
      n297 = Add(x=w271, y="Aj 7-1") -> (x+y=w535:dbl)
      "B 7-1" <- w535
      n298 = Add(x=w269, y="Aj7+1") -> (x+y=w509:dbl)
      "B7+1" <- w509
      n299 = Less?(x=w466, y=w474) -> (x < y?=w473:bool)
      n300 = Add(x=w174, y="Aj 21+1") -> (x+y=w165:dbl)
      "B  21+1" <- w165
      n301 = Add(x=w176, y="Aj 21") -> (x+y=w185:dbl)
      "B  21" <- w185
      n302 = Greater?(x=w490, y=w495) -> (0:w496:bool)
      n303 = And(x=w418, y=w417) -> (x .and. y?=w415:bool)
      n304 = Add(x=w196, y="Aj 21-1") -> (x+y=w186:dbl)
      "B  21-1" <- w186
      n305 = Subtract(x=w422, y=w416) -> (x-y=w414:dbl)
      n306 = And(x=w396, y=w395) -> (x .and. y?=w393:bool)
      n307 = Subtract(x=w399, y=w394) -> (x-y=w392:dbl)
      n308 = feedback #36() -> (w238:dbl)  [unwired: 1 in]
      "B18-1" <- w238
      n309 = case shown="True" "Baseline" {
        tunnel: w229 -> [_ w671]
        tunnel: [w670 w671] -> w230
        tunnel: w238 -> [w670 _]
        frame False {
        }
        frame True {
        }
      }
      n310 = feedback-in #36(w230) -> ()
      n311 = And(x=w404, y=w405) -> (x .and. y?=w407:bool)
      n312 = Less?(x=w490, y=w498) -> (x < y?=w497:bool)
      n313 = And(x=w429, y=w430) -> (x .and. y?=w432:bool)
      n314 = Subtract(x=w401, y=w406) -> (x-y=w408:dbl)
      n315 = Subtract(x=w424, y=w431) -> (x-y=w433:dbl)
      n316 = Greater?(x=w133, y=w143) -> (0:w138:bool)
      n317 = Greater?(x=w145, y=w144) -> (0:w150:bool)
      n318 = Multiply(x=w174, y=4.0) -> (x*y=w172:dbl)
      "N21+1" <- w172
      n319 = And(x=w443, y=w442) -> (x .and. y?=w440:bool)
      n320 = Less?(x=w133, y=w136) -> (x < y?=w137:bool)
      n321 = Subtract(x=w446, y=w441) -> (x-y=w439:dbl)
      n322 = Multiply(x=w269, y=4.0) -> (x*y=w512:dbl)
      "N7+1" <- w512
      n323 = Less?(x=w145, y=w152) -> (x < y?=w151:bool)
      n324 = Multiply(x=w270, y=4.0) -> (x*y=w525:dbl)
      "N7" <- w525
      n325 = And(x=w452, y=w453) -> (x .and. y?=w455:bool)
      n326 = Subtract(x=w447, y=w454) -> (x-y=w456:dbl)
      n327 = Greater?(x=w477, y=w483) -> (0:w484:bool)
      n328 = Less?(x=w121, y=w130) -> (x < y?=w129:bool)
      n329 = Add(x=w274, y="Aj 12-1") -> (x+y=w557:dbl)
      "B 12-1" <- w557
      n330 = Multiply(x=w176, y=4.0) -> (x*y=w178:dbl)
      "N21" <- w178
      n331 = Less?(x=w477, y=w486) -> (x < y?=w485:bool)
      n332 = Multiply(x=w271, y=4.0) -> (x*y=w538:dbl)
      "N7-1" <- w538
      n333 = Add(x=w275, y="Aj 6+1") -> (x+y=w588:dbl)
      "B 6+1" <- w588
      n334 = And(x=w473, y=w472) -> (x .and. y?=w470:bool)
      n335 = Multiply(x=w196, y=4.0) -> (x*y=w194:dbl)
      "N21-1" <- w194
      n336 = Subtract(x=w466, y=w471) -> (x-y=w469:dbl)
      n337 = Add(x=w272, y="Aj 12+1") -> (x+y=w575:dbl)
      "B 12+1" <- w575
      n338 = Greater?(x=w121, y=w123) -> (0:w128:bool)
      n339 = Add(x=w276, y="Aj 6") -> (x+y=w601:dbl)
      "B6" <- w601
      n340 = Add(x=w277, y="Aj 6-1") -> (x+y=w615:dbl)
      "B 6-1" <- w615
      n341 = Add(x=w273, y="Aj 12") -> (x+y=w566:dbl)
      "B12" <- w566
      n342 = And(x=w497, y=w496) -> (x .and. y?=w494:bool)
      n343 = Subtract(x=w490, y=w495) -> (x-y=w493:dbl)
      n344 = And(x=w137, y=w138) -> (x .and. y?=w139:bool)
      n345 = Multiply(x=w274, y=4.0) -> (x*y=w554:dbl)
      "N12-1" <- w554
      n346 = Subtract(x=w133, y=w143) -> (x-y=w140:dbl)
      n347 = Multiply(x=w275, y=4.0) -> (x*y=w591:dbl)
      "N6+1" <- w591
      n348 = Add(x=w215, y="Aj 18+1") -> (x+y=w206:dbl)
      "B  18+1" <- w206
      n349 = Add(x=w218, y="Aj 18") -> (x+y=w227:dbl)
      "B  18" <- w227
      n350 = Greater?(x=w514, y=w522) -> (0:w523:bool)
      n351 = And(x=w151, y=w150) -> (x .and. y?=w149:bool)
      n352 = Add(x=w238, y="Aj 18-1") -> (x+y=w228:dbl)
      "B  18-1" <- w228
      n353 = And(x=w129, y=w128) -> (x .and. y?=w127:bool)
      n354 = And(x=w485, y=w484) -> (x .and. y?=w482:bool)
      n355 = Greater?(x=w517, y=w535) -> (0:w536:bool)
      n356 = Subtract(x=w477, y=w483) -> (x-y=w481:dbl)
      n357 = Less?(x=w514, y=w525) -> (x < y?=w524:bool)
      n358 = Multiply(x=w272, y=4.0) -> (x*y=w572:dbl)
      "N12+1" <- w572
      n359 = Less?(x=w517, y=w538) -> (x < y?=w537:bool)
      n360 = Subtract(x=w145, y=w144) -> (x-y=w148:dbl)
      n361 = Multiply(x=w276, y=4.0) -> (x*y=w598:dbl)
      "N6" <- w598
      n362 = Subtract(x=w121, y=w123) -> (x-y=w126:dbl)
      n363 = Multiply(x=w277, y=4.0) -> (x*y=w618:dbl)
      "N6-1" <- w618
      n364 = Multiply(x=w215, y=4.0) -> (x*y=w213:dbl)
      "N18+1" <- w213
      n365 = Greater?(x=w175, y=w185) -> (0:w180:bool)
      n366 = Greater?(x=w503, y=w509) -> (0:w510:bool)
      n367 = Greater?(x=w187, y=w186) -> (0:w192:bool)
      n368 = Less?(x=w503, y=w512) -> (x < y?=w511:bool)
      n369 = case shown="True" w91 {
        tunnel: w92 -> [_ w629]
        tunnel: [0.0 w629] -> w67
        frame False {
        }
        frame True {
        }
      }
      n370 = Less?(x=w175, y=w178) -> (x < y?=w179:bool)
      n371 = Multiply(x=w273, y=4.0) -> (x*y=w569:dbl)
      "N12" <- w569
      n372 = case shown="True" w79 {
        tunnel: w78 -> [_ w633]
        tunnel: [0.0 w633] -> w68
        frame False {
        }
        frame True {
        }
      }
      n373 = case shown="True" w99 {
        tunnel: w98 -> [_ w625]
        tunnel: [0.0 w625] -> w66
        frame False {
        }
        frame True {
        }
      }
      n374 = Less?(x=w187, y=w194) -> (x < y?=w193:bool)
      n375 = Multiply(x=w218, y=4.0) -> (x*y=w220:dbl)
      "N18" <- w220
      n376 = Less?(x=w163, y=w172) -> (x < y?=w171:bool)
      n377 = Greater?(x=w549, y=w557) -> (0:w556:bool)
      n378 = Multiply(x=w238, y=4.0) -> (x*y=w236:dbl)
      "N18-1" <- w236
      n379 = Greater?(x=w581, y=w588) -> (0:w589:bool)
      n380 = Less?(x=w549, y=w554) -> (x < y?=w555:bool)
      n381 = case shown="True" w318 {
        tunnel: w317 -> [_ w679]
        tunnel: [0.0 w679] -> w298
        frame False {
        }
        frame True {
        }
      }
      n382 = case shown="True" w332 {
        tunnel: w333 -> [_ w683]
        tunnel: [0.0 w683] -> w299
        frame False {
        }
        frame True {
        }
      }
      n383 = case shown="True" w308 {
        tunnel: w309 -> [_ w675]
        tunnel: [0.0 w675] -> w297
        frame False {
        }
        frame True {
        }
      }
      n384 = Less?(x=w581, y=w591) -> (x < y?=w590:bool)
      n385 = Greater?(x=w163, y=w165) -> (0:w170:bool)
      n386 = And(x=w524, y=w523) -> (x .and. y?=w521:bool)
      n387 = Subtract(x=w514, y=w522) -> (x-y=w520:dbl)
      n388 = Greater?(x=w542, y=w575) -> (0:w574:bool)
      n389 = And(x=w537, y=w536) -> (x .and. y?=w534:bool)
      n390 = And(x=w511, y=w510) -> (x .and. y?=w508:bool)
      n391 = Subtract(x=w517, y=w535) -> (x-y=w533:dbl)
      n392 = Greater?(x=w595, y=w601) -> (0:w600:bool)
      n393 = Less?(x=w542, y=w572) -> (x < y?=w573:bool)
      n394 = Greater?(x=w614, y=w615) -> (0:w616:bool)
      n395 = Subtract(x=w503, y=w509) -> (x-y=w507:dbl)
      n396 = And(x=w179, y=w180) -> (x .and. y?=w181:bool)
      n397 = Less?(x=w595, y=w598) -> (x < y?=w599:bool)
      n398 = Less?(x=w614, y=w618) -> (x < y?=w617:bool)
      n399 = Greater?(x=w546, y=w566) -> (0:w567:bool)
      n400 = Subtract(x=w175, y=w185) -> (x-y=w182:dbl)
      n401 = case shown="True" w359 {
        tunnel: w358 -> [_ w691]
        tunnel: [0.0 w691] -> w338
        frame False {
        }
        frame True {
        }
      }
      n402 = Less?(x=w546, y=w569) -> (x < y?=w568:bool)
      n403 = case shown="True" w139 {
        tunnel: w140 -> [_ w641]
        tunnel: [0.0 w641] -> w112
        frame False {
        }
        frame True {
        }
      }
      n404 = case shown="True" w370 {
        tunnel: w369 -> [_ w695]
        tunnel: [0.0 w695] -> w339
        frame False {
        }
        frame True {
        }
      }
      n405 = And(x=w193, y=w192) -> (x .and. y?=w191:bool)
      n406 = And(x=w171, y=w170) -> (x .and. y?=w169:bool)
      n407 = case shown="True" w346 {
        tunnel: w345 -> [_ w687]
        tunnel: [0.0 w687] -> w337
        frame False {
        }
        frame True {
        }
      }
      n408 = case shown="True" w149 {
        tunnel: w148 -> [_ w645]
        tunnel: [0.0 w645] -> w113
        frame False {
        }
        frame True {
        }
      }
      n409 = case shown="True" w127 {
        tunnel: w126 -> [_ w637]
        tunnel: [0.0 w637] -> w111
        frame False {
        }
        frame True {
        }
      }
      n410 = Greater?(x=w216, y=w227) -> (0:w222:bool)
      n411 = Greater?(x=w229, y=w228) -> (0:w234:bool)
      n412 = Subtract(x=w187, y=w186) -> (x-y=w190:dbl)
      n413 = Subtract(x=w163, y=w165) -> (x-y=w168:dbl)
      n414 = Less?(x=w216, y=w220) -> (x < y?=w221:bool)
      n415 = And(x=w555, y=w556) -> (x .and. y?=w558:bool)
      n416 = Subtract(x=w549, y=w557) -> (x-y=w559:dbl)
      n417 = Less?(x=w229, y=w236) -> (x < y?=w235:bool)
      n418 = Subtract(x=w581, y=w588) -> (x-y=w586:dbl)
      n419 = Less?(x=w202, y=w213) -> (x < y?=w212:bool)
      n420 = case shown="True" w415 {
        tunnel: w414 -> [_ w707]
        tunnel: [0.0 w707] -> w378
        frame False {
        }
        frame True {
        }
      }
      n421 = case shown="True" w393 {
        tunnel: w392 -> [_ w699]
        tunnel: [0.0 w699] -> w376
        frame False {
        }
        frame True {
        }
      }
      n422 = And(x=w590, y=w589) -> (x .and. y?=w587:bool)
      n423 = case shown="True" w407 {
        tunnel: w408 -> [_ w703]
        tunnel: [0.0 w703] -> w377
        frame False {
        }
        frame True {
        }
      }
      n424 = case shown="True" w432 {
        tunnel: w433 -> [_ w711]
        tunnel: [0.0 w711] -> w379
        frame False {
        }
        frame True {
        }
      }
      n425 = case shown="True" w440 {
        tunnel: w439 -> [_ w715]
        tunnel: [0.0 w715] -> w380
        frame False {
        }
        frame True {
        }
      }
      n426 = And(x=w617, y=w616) -> (x .and. y?=w613:bool)
      n427 = Subtract(x=w595, y=w601) -> (x-y=w603:dbl)
      n428 = And(x=w573, y=w574) -> (x .and. y?=w576:bool)
      n429 = Subtract(x=w614, y=w615) -> (x-y=w612:dbl)
      n430 = case shown="True" w455 {
        tunnel: w456 -> [_ w719]
        tunnel: [0.0 w719] -> w381
        frame False {
        }
        frame True {
        }
      }
      n431 = And(x=w599, y=w600) -> (x .and. y?=w602:bool)
      n432 = Greater?(x=w202, y=w206) -> (0:w211:bool)
      n433 = Subtract(x=w546, y=w566) -> (x-y=w564:dbl)
      n434 = Subtract(x=w542, y=w575) -> (x-y=w577:dbl)
      n435 = And(x=w568, y=w567) -> (x .and. y?=w565:bool)
      n436 = case shown="True" w169 {
        tunnel: w168 -> [_ w649]
        tunnel: [0.0 w649] -> w156
        frame False {
        }
        frame True {
        }
      }
      n437 = And(x=w221, y=w222) -> (x .and. y?=w223:bool)
      n438 = case shown="True" w191 {
        tunnel: w190 -> [_ w657]
        tunnel: [0.0 w657] -> w158
        frame False {
        }
        frame True {
        }
      }
      n439 = case shown="True" w470 {
        tunnel: w469 -> [_ w723]
        tunnel: [0.0 w723] -> w461
        frame False {
        }
        frame True {
        }
      }
      n440 = Subtract(x=w216, y=w227) -> (x-y=w224:dbl)
      n441 = case shown="True" w482 {
        tunnel: w481 -> [_ w727]
        tunnel: [0.0 w727] -> w462
        frame False {
        }
        frame True {
        }
      }
      n442 = case shown="True" w521 {
        tunnel: w520 -> [_ w739]
        tunnel: [0.0 w739] -> w501
        frame False {
        }
        frame True {
        }
      }
      n443 = case shown="True" w494 {
        tunnel: w493 -> [_ w731]
        tunnel: [0.0 w731] -> w463
        frame False {
        }
        frame True {
        }
      }
      n444 = And(x=w235, y=w234) -> (x .and. y?=w233:bool)
      n445 = case shown="True" w181 {
        tunnel: w182 -> [_ w653]
        tunnel: [0.0 w653] -> w157
        frame False {
        }
        frame True {
        }
      }
      n446 = And(x=w212, y=w211) -> (x .and. y?=w210:bool)
      n447 = case shown="False" w534 {
        tunnel: w533 -> [_ w743]
        tunnel: [0.0 w743] -> w527
        frame False {
        }
        frame True {
        }
      }
      n448 = case shown="True" w508 {
        tunnel: w507 -> [_ w735]
        tunnel: [0.0 w735] -> w500
        frame False {
        }
        frame True {
        }
      }
      n449 = Subtract(x=w229, y=w228) -> (x-y=w232:dbl)
      n450 = Subtract(x=w202, y=w206) -> (x-y=w209:dbl)
      n451 = case shown="True" w565 {
        tunnel: w564 -> [_ w751]
        tunnel: [0.0 w751] -> w541
        frame False {
        }
        frame True {
        }
      }
      n452 = case shown="True" w558 {
        tunnel: w559 -> [_ w755]
        tunnel: [0.0 w755] -> w548
        frame False {
        }
        frame True {
        }
      }
      n453 = case shown="True" w576 {
        tunnel: w577 -> [_ w747]
        tunnel: [0.0 w747] -> w540
        frame False {
        }
        frame True {
        }
      }
      n454 = case shown="True" w587 {
        tunnel: w586 -> [_ w759]
        tunnel: [0.0 w759] -> w580
        frame False {
        }
        frame True {
        }
      }
      n455 = case shown="True" w613 {
        tunnel: w612 -> [_ w767]
        tunnel: [0.0 w767] -> w610
        frame False {
        }
        frame True {
        }
      }
      n456 = case shown="True" w602 {
        tunnel: w603 -> [_ w763]
        tunnel: [0.0 w763] -> w593
        frame False {
        }
        frame True {
        }
      }
      n457 = case shown="True" w223 {
        tunnel: w224 -> [_ w665]
        tunnel: [0.0 w665] -> w200
        frame False {
        }
        frame True {
        }
      }
      n458 = case shown="True" w233 {
        tunnel: w232 -> [_ w669]
        tunnel: [0.0 w669] -> w201
        frame False {
        }
        frame True {
        }
      }
      n459 = case shown="True" w210 {
        tunnel: w209 -> [_ w661]
        tunnel: [0.0 w661] -> w199
        frame False {
        }
        frame True {
        }
      }
      n460 = Build Array(w527, w501, w500, w463, w462, w461, w158, w157, w156) -> (w528:dbl[])
      "7 Hz" <- w528
      n461 = Array Max & Min(array=w528) -> (max value=w296:dbl, max index (indices)=→"Max Index 7":i32)  [unwired: 2 out]
      "PSD max 7" <- w296
      n462 = Build Array(w610, w593, w580, w548, w541, w540, w201, w200, w199) -> (w608:dbl[])
      "6 Hz" <- w608
      n463 = Build Array(w381, w380, w379, w378, w377, w376, w113, w112, w111) -> (w382:dbl[])
      "8 Hz" <- w382
      n464 = Build Array(w339, w338, w337, w299, w298, w297, w68, w67, w66) -> (w340:dbl[])
      "11 Hz" <- w340
      n465 = Array Max & Min(array=w608) -> (max value=w293:dbl, max index (indices)=→"Max Index 6":i32)  [unwired: 2 out]
      "PSD max 6" <- w293
      n466 = Array Max & Min(array=w382) -> (max value=w295:dbl, max index (indices)=→"Max Index 8":i32)  [unwired: 2 out]
      "PSD max 8" <- w295
      n467 = Array Max & Min(array=w340) -> (max value=w294:dbl, max index (indices)=→"Max Index 11":i32)  [unwired: 2 out]
      "PSD max 11" <- w294
      n468 = Build Array(w293, w296, w295, w294) -> (w292:dbl[])
      n469 = Array Max & Min(array=w292) -> (max value=w290:dbl, max index (indices)=w291:i32)  [unwired: 2 out]
      "max value" <- w290
      "PSD MAX" <- w290
      n470 = Greater?(x=w290, y=0.0 ("x")) -> (0:w288:bool)
      n471 = case shown="True" w288 {
        tunnel: w291 -> [_ w673]
        tunnel: [555 w673] -> w280
        frame False {
        }
        frame True {
        }
      }
      "Index ที่มากที่สุด" <- w280
      n472 = Equal?(x=0, y=w280) -> (x = y?=→"6 HZ":bool)
      n473 = Equal?(x=1, y=w280) -> (x = y?=→"7 HZ":bool)
      n474 = Equal?(x=2, y=w280) -> (x = y?=→"8 HZ":bool)
      n475 = Equal?(x=3, y=w280) -> (x = y?=→"11 HZ":bool)
      n476 = Equal?(x=555, y=w280) -> (x = y?=→"555":bool)
    }
  }
  n477 = while {
    shift-right: [w779] -> _
    shift-left: "" -> [w781]
    stop <- FALSE stop-if-true
    n478 = event shown="[3] \"call_back\": Value Change" {
      selector: _ -> [_ _ _ _]
      dyn-events: _ -> [_ _ _ _]
      timeout: _ -> [_ _ _ _]
      tunnel: w781 -> [_ _ _ _]
      tunnel: ["0622436287" "1669" " 0937529340" _] -> w779
      event Value Change {
        n479 = event-data() -> ()  [unwired: 1 in, 6 out]
      }
      event "1": Value Change {
        n480 = event-data() -> ()  [unwired: 1 in, 6 out]
      }
      event "1 3": Value Change {
        n481 = event-data() -> ()  [unwired: 1 in, 6 out]
      }
      event "call_back": Value Change {
        n482 = event-data() -> ()  [unwired: 1 in, 6 out]
        n483 = local write "Tab Control"(enum32{"TAB 1", "TAB 2", "TAB 3", "TAB 4"}."TAB 1" ("Tab Control")) -> ()
      }
    }
    "String 2" <- w779
  }
  n484 = while {
    stop <- FALSE stop-if-true
    n485 = while {
      stop <- FALSE stop-if-true
      n486 = while {
        stop <- FALSE stop-if-true
        w825 = 66.666667
        # "6 HZ"
        n487 = for {
          N: 2 -> [_]
          tunnel: w825 -> [w829]
          i -> [w831]
          n488 = Wait (ms)(milliseconds to wait=w829) -> ()  [unwired: 1 out]
          n489 = Equal?(x=0, y=w831) -> (x = y?=→"?" →"?" →"?" →"?" →"?" →"?" →"?" →"?" →"?" →"?":bool)
        }
        n490 = for {
          N: 2 -> [_]
          tunnel: w825 -> [w833]
          i -> [w834]
          n491 = Wait (ms)(milliseconds to wait=w833) -> ()  [unwired: 1 out]
          n492 = Equal?(x=1, y=w834) -> (x = y?=→"?" →"?" →"?" →"?" →"?" →"?" →"?" →"?" →"?" →"?":bool)
        }
      }
      n493 = while {
        stop <- FALSE stop-if-true
        w813 = 57.142857
        # "7 HZ"
        n494 = for {
          N: 2 -> [_]
          tunnel: w813 -> [w817]
          i -> [w819]
          n495 = Wait (ms)(milliseconds to wait=w817) -> ()  [unwired: 1 out]
          n496 = Equal?(x=0, y=w819) -> (x = y?=→"?" →"?" →"?" →"?" →"?" →"?" →"?" →"?" →"?" →"?":bool)
        }
        n497 = for {
          N: 2 -> [_]
          tunnel: w813 -> [w821]
          i -> [w822]
          n498 = Wait (ms)(milliseconds to wait=w821) -> ()  [unwired: 1 out]
          n499 = Equal?(x=1, y=w822) -> (x = y?=→"?" →"?" →"?" →"?" →"?" →"?" →"?" →"?" →"?" →"?":bool)
        }
      }
      n500 = while {
        stop <- FALSE stop-if-true
        w801 = 36.3636363636
        # "11 36.36363636"
        # "11 HZ"
        n501 = for {
          N: 2 -> [_]
          tunnel: w801 -> [w805]
          i -> [w807]
          n502 = Wait (ms)(milliseconds to wait=w805) -> ()  [unwired: 1 out]
          n503 = Equal?(x=0, y=w807) -> (x = y?=→"?" →"?" →"?" →"?" →"?" →"?" →"?" →"?" →"?" →"?":bool)
        }
        n504 = for {
          N: 2 -> [_]
          tunnel: w801 -> [w809]
          i -> [w810]
          n505 = Wait (ms)(milliseconds to wait=w809) -> ()  [unwired: 1 out]
          n506 = Equal?(x=1, y=w810) -> (x = y?=→"?" →"?" →"?" →"?" →"?" →"?" →"?" →"?" →"?" →"?":bool)
        }
      }
      n507 = while {
        stop <- FALSE stop-if-true
        w789 = 50.0
        # "8 HZ"
        n508 = for {
          N: 2 -> [_]
          tunnel: w789 -> [w793]
          i -> [w795]
          n509 = Wait (ms)(milliseconds to wait=w793) -> ()  [unwired: 1 out]
          n510 = Equal?(x=0, y=w795) -> (x = y?=→"?" →"?" →"?" →"?" →"?" →"?" →"?" →"?" →"?" →"?":bool)
        }
        n511 = for {
          N: 2 -> [_]
          tunnel: w789 -> [w797]
          i -> [w798]
          n512 = Wait (ms)(milliseconds to wait=w797) -> ()  [unwired: 1 out]
          n513 = Equal?(x=1, y=w798) -> (x = y?=→"?" →"?" →"?" →"?" →"?" →"?" →"?" →"?" →"?" →"?":bool)
        }
      }
    }
  }
  n514 = while {
    stop <- FALSE stop-if-true
    n515 = event shown="[4] \"Emer\": Value Change" {
      selector: _ -> [_ _ _ _ _ _ _]
      dyn-events: _ -> [_ _ _ _ _ _ _]
      timeout: _ -> [_ _ _ _ _ _ _]
      event Timeout {
        n516 = event-data() -> ()  [unwired: 1 in, 3 out]
      }
      event Value Change {
        n517 = event-data() -> ()  [unwired: 1 in, 6 out]
        n518 = local write "Tab Control"(enum32{"TAB 1", "TAB 2", "TAB 3", "TAB 4"}."TAB 2" ("Tab Control")) -> ()
      }
      event Value Change {
        n519 = event-data() -> ()  [unwired: 1 in, 6 out]
        n520 = local write "Tab Control"(enum32{"TAB 1", "TAB 2", "TAB 3", "TAB 4"}."TAB 3" ("Tab Control")) -> ()
      }
      event Value Change {
        n521 = event-data() -> ()  [unwired: 1 in, 6 out]
        n522 = local write "Tab Control"(T9."TAB 1" ("Tab Control")) -> ()
      }
      event "Emer": Value Change {
        n523 = event-data() -> ()  [unwired: 1 in, 6 out]
        n524 = local write "Tab Control"(enum32{"TAB 1", "TAB 2", "TAB 3", "TAB 4"}."TAB 4" ("Tab Control")) -> ()
      }
      event Value Change {
        n525 = event-data() -> ()  [unwired: 1 in, 6 out]
        n526 = local write "Tab Control"(enum32{"TAB 1", "TAB 2", "TAB 3", "TAB 4"}."TAB 4" ("Tab Control")) -> ()
      }
      event "BACK_Page4": Value Change {
        n527 = event-data() -> ()  [unwired: 1 in, 6 out]
        n528 = local write "Tab Control"(enum32{"TAB 1", "TAB 2", "TAB 3", "TAB 4"}."TAB 1" ("Tab Control")) -> ()
      }
    }
  }
  n529 = local read "Tab Control"() -> (w2:enum32{"TAB 1", "TAB 2", "TAB 3", "TAB 4"})
  n530 = Obtain Notifier(notification data type=w2) -> (notifier out=w1:refnum<notifier>, error out=w4:errorcluster)  [unwired: 3 in, 1 out]
  n531 = while {
    tunnel: w1 -> [w844]
    stop <- FALSE stop-if-true
    n532 = Wait on Notification(notifier=w844) -> (notification=w843:enum32{"TAB 1", "TAB 2", "TAB 3", "TAB 4"})  [unwired: 3 in, 3 out]
    n533 = case shown="\"TAB 4\"" w843 {
      frame "TAB 1" {
        n534 = while {
          stop <- w875 stop-if-true
          n535 = local read "Baseline"() -> (w867:bool)
          n536 = case shown="False" w867 {
            tunnel: ["start" FALSE] -> w866
            frame False {
            }
            frame True {
            }
          }
          n537 = feedback #37() -> (w887:i32)  [unwired: 1 in]
          n538 = case shown="True" w866 {
            tunnel: [w913 w914] -> w888
            tunnel: w887 -> [w913 w915]
            frame False {
            }
            frame True {
              n539 = Increment(x=w915) -> (x+1=w914:i32)
            }
          }
          n540 = case shown="3" w888 {
            selector: w888 -> [w892 w896 w897 w904 w908 w911]
            tunnel: [w892 w896 w897 w904 w908 w910] -> w886
            frame 0, Default {
              w891 = FALSE ("B")
              n541 = local write "ele"(w891) -> ()
              n542 = local write "call"(w891) -> ()
              n543 = local write "commu"(w891) -> ()
              n544 = local write "Emotion"(w891) -> ()
              n545 = local write "Activity"(w891) -> ()
              n546 = local write "ACC"(w891) -> ()
            }
            frame 1 {
              n547 = local write "Emer"(FALSE) -> ()
              n548 = Wait (ms)(milliseconds to wait=u32 1500 ("millisecond timer value")) -> ()  [unwired: 1 out]
              "ele" <- TRUE
            }
            frame 2 {
              n549 = local write "ele"(FALSE) -> ()
              n550 = Wait (ms)(milliseconds to wait=u32 1000) -> ()  [unwired: 1 out]
              "call" <- TRUE
            }
            frame 3 {
              n551 = local write "call"(FALSE) -> ()
              n552 = Wait (ms)(milliseconds to wait=u32 1000) -> ()  [unwired: 1 out]
              "commu" <- TRUE
            }
            frame 4 {
              n553 = local write "commu"(FALSE) -> ()
              n554 = Wait (ms)(milliseconds to wait=u32 1000) -> ()  [unwired: 1 out]
              "Emer" <- TRUE
            }
            frame 5 {
              n555 = Subtract(x=w911, y=5 ("x")) -> (x-y=w910:i32)
              n556 = Wait (ms)(milliseconds to wait=u32 1200 ("millisecond timer value")) -> ()  [unwired: 1 out]
            }
          }
          n557 = feedback-in #37(w886) -> ()
          n558 = local read "Tab Control"() -> (w877:enum32{"TAB 1", "TAB 2", "TAB 3", "TAB 4"})
          n559 = Equal?(x=w877, y=T9."TAB 2" ("Tab Control")) -> (x = y?=w885:bool)
          n560 = Equal?(x=w877, y=T9."TAB 6" ("Tab Control")) -> (x = y?=w879:bool)
          n561 = Equal?(x=w877, y=T9."TAB 3" ("Tab Control")) -> (x = y?=w884:bool)
          n562 = Equal?(x=w877, y=T9."TAB 4" ("Tab Control")) -> (x = y?=w883:bool)
          n563 = Equal?(x=w877, y=T9."TAB 7" ("Tab Control")) -> (x = y?=w878:bool)
          n564 = Equal?(x=w877, y=T9."TAB 5" ("Tab Control")) -> (x = y?=w882:bool)
          n565 = Or(x=w885, y=w884) -> (x .or. y?=w881:bool)
          n566 = Or(x=w879, y=w878) -> (x .or. y?=w874:bool)
          n567 = Or(x=w883, y=w882) -> (x .or. y?=w880:bool)
          n568 = Or(x=w881, y=w880) -> (x .or. y?=w876:bool)
          n569 = Or(x=w876, y=w874) -> (x .or. y?=w875:bool)
        }
        n570 = while {
          stop <- w847 stop-if-true
          w846 = FALSE
          n571 = local read "Tab Control"() -> (w857:enum32{"TAB 1", "TAB 2", "TAB 3", "TAB 4"})
          n572 = Equal?(x=w857, y=T9."TAB 2" ("Tab Control")) -> (x = y?=w865:bool)
          n573 = Equal?(x=w857, y=T9."TAB 3" ("Tab Control")) -> (x = y?=w864:bool)
          n574 = Equal?(x=w857, y=T9."TAB 4" ("Tab Control")) -> (x = y?=w863:bool)
          n575 = Equal?(x=w857, y=T9."TAB 5" ("Tab Control")) -> (x = y?=w853:bool)
          n576 = Equal?(x=w857, y=T9."TAB 6" ("Tab Control")) -> (x = y?=w852:bool)
          n577 = Equal?(x=w857, y=T9."TAB 7" ("Tab Control")) -> (x = y?=w849:bool)
          n578 = Or(x=w865, y=w864) -> (x .or. y?=w862:bool)
          n579 = Or(x=w864, y=w863) -> (x .or. y?=w861:bool)
          n580 = Or(x=w853, y=w852) -> (x .or. y?=w850:bool)
          n581 = Or(x=w862, y=w861) -> (x .or. y?=w851:bool)
          n582 = Or(x=w850, y=w849) -> (x .or. y?=w848:bool)
          n583 = Or(x=w851, y=w848) -> (x .or. y?=w847:bool)
          "Clear1" <- w847
          n584 = local write "Clear2"(w846) -> ()
          n585 = local write "Clear 3"(w846) -> ()
          n586 = local write "Clear4"(w846) -> ()
        }
      }
      frame "TAB 2" {
        n587 = while {
          stop <- w944 stop-if-true
          n588 = local read "start"() -> (w936:bool)
          n589 = feedback #38() -> (w956:i32)  [unwired: 1 in]
          n590 = case shown="True" w936 {
            tunnel: [w980 w981] -> w957
            tunnel: w956 -> [w980 w982]
            frame False {
            }
            frame True {
              n591 = Increment(x=w982) -> (x+1=w981:i32)
            }
          }
          n592 = case shown="0, Default" w957 {
            selector: w957 -> [w959 w963 w966 w971 w975 w978]
            tunnel: [w959 w963 w966 w971 w975 w977] -> w955
            frame 0, Default {
              w958 = FALSE ("B")
              n593 = local write "Activity"(w958) -> ()
              n594 = local write "Emotion"(w958) -> ()
              n595 = local write "back_page2"(w958) -> ()
              n596 = local write "ACC"(w958) -> ()
            }
            frame 1 {
              w961 = TRUE
              n597 = local write "back_page2"(FALSE) -> ()
              n598 = Wait (ms)(milliseconds to wait=u32 1500 ("millisecond timer value")) -> ()  [unwired: 1 out]
              "commu_1" <- w961
              "Activity" <- w961
            }
            frame 2 {
              w965 = TRUE
              n599 = local write "Activity"(FALSE) -> ()
              n600 = Wait (ms)(milliseconds to wait=u32 1000) -> ()  [unwired: 1 out]
              "commu_2" <- w965
              "Emotion" <- w965
            }
            frame 3 {
              w969 = TRUE
              n601 = local write "Emotion"(FALSE) -> ()
              n602 = Wait (ms)(milliseconds to wait=u32 1000) -> ()  [unwired: 1 out]
              "8-2" <- w969
              "ACC" <- w969
            }
            frame 4 {
              w972 = TRUE
              n603 = local write "ACC"(FALSE) -> ()
              n604 = Wait (ms)(milliseconds to wait=u32 1000) -> ()  [unwired: 1 out]
              "commu_back" <- w972
              "back_page2" <- w972
            }
            frame 5 {
              n605 = Subtract(x=w978, y=5 ("x")) -> (x-y=w977:i32)
              n606 = Wait (ms)(milliseconds to wait=u32 1200 ("millisecond timer value")) -> ()  [unwired: 1 out]
            }
          }
          n607 = feedback-in #38(w955) -> ()
          n608 = local read "Tab Control"() -> (w946:enum32{"TAB 1", "TAB 2", "TAB 3", "TAB 4"})
          n609 = Equal?(x=w946, y=T9."TAB 1" ("Tab Control")) -> (x = y?=w954:bool)
          n610 = Equal?(x=w946, y=T9."TAB 6" ("Tab Control")) -> (x = y?=w948:bool)
          n611 = Equal?(x=w946, y=T9."TAB 3" ("Tab Control")) -> (x = y?=w953:bool)
          n612 = Equal?(x=w946, y=T9."TAB 4" ("Tab Control")) -> (x = y?=w952:bool)
          n613 = Equal?(x=w946, y=T9."TAB 7" ("Tab Control")) -> (x = y?=w947:bool)
          n614 = Equal?(x=w946, y=T9."TAB 5" ("Tab Control")) -> (x = y?=w951:bool)
          n615 = Or(x=w954, y=w953) -> (x .or. y?=w950:bool)
          n616 = Or(x=w948, y=w947) -> (x .or. y?=w943:bool)
          n617 = Or(x=w952, y=w951) -> (x .or. y?=w949:bool)
          n618 = Or(x=w950, y=w949) -> (x .or. y?=w945:bool)
          n619 = Or(x=w945, y=w943) -> (x .or. y?=w944:bool)
        }
        n620 = while {
          stop <- w917 stop-if-true
          w916 = FALSE
          n621 = local read "Tab Control"() -> (w927:enum32{"TAB 1", "TAB 2", "TAB 3", "TAB 4"})
          n622 = Equal?(x=w927, y=T9."TAB 1" ("Tab Control")) -> (x = y?=w935:bool)
          n623 = Equal?(x=w927, y=T9."TAB 3" ("Tab Control")) -> (x = y?=w934:bool)
          n624 = Equal?(x=w927, y=T9."TAB 4" ("Tab Control")) -> (x = y?=w933:bool)
          n625 = Equal?(x=w927, y=T9."TAB 5" ("Tab Control")) -> (x = y?=w923:bool)
          n626 = Equal?(x=w927, y=T9."TAB 6" ("Tab Control")) -> (x = y?=w922:bool)
          n627 = Equal?(x=w927, y=T9."TAB 7" ("Tab Control")) -> (x = y?=w919:bool)
          n628 = Or(x=w935, y=w934) -> (x .or. y?=w932:bool)
          n629 = Or(x=w934, y=w933) -> (x .or. y?=w931:bool)
          n630 = Or(x=w923, y=w922) -> (x .or. y?=w920:bool)
          n631 = Or(x=w932, y=w931) -> (x .or. y?=w921:bool)
          n632 = Or(x=w920, y=w919) -> (x .or. y?=w918:bool)
          n633 = Or(x=w921, y=w918) -> (x .or. y?=w917:bool)
          "Clear2" <- w917
          n634 = local write "Clear 3"(w916) -> ()
          n635 = local write "Clear1"(w916) -> ()
          n636 = local write "Clear4"(w916) -> ()
        }
      }
      frame "TAB 3" {
        n637 = while {
          stop <- w1011 stop-if-true
          n638 = local read "start"() -> (w1003:bool)
          n639 = feedback #39() -> (w1023:i32)  [unwired: 1 in]
          n640 = case shown="True" w1003 {
            tunnel: [w1047 w1048] -> w1024
            tunnel: w1023 -> [w1047 w1049]
            frame False {
            }
            frame True {
              n641 = Increment(x=w1049) -> (x+1=w1048:i32)
            }
          }
          n642 = case shown="5" w1024 {
            selector: w1024 -> [w1026 w1030 w1033 w1038 w1042 w1045]
            tunnel: [w1026 w1030 w1033 w1038 w1042 w1044] -> w1022
            frame 0, Default {
              w1025 = FALSE ("B")
              n643 = local write "call_back"(w1025) -> ()
              n644 = local write "call_1"(w1025) -> ()
              n645 = local write "call_2"(w1025) -> ()
              n646 = local write "call_3"(w1025) -> ()
            }
            frame 1 {
              w1027 = TRUE
              n647 = local write "call_back"(FALSE) -> ()
              n648 = Wait (ms)(milliseconds to wait=u32 1500 ("millisecond timer value")) -> ()  [unwired: 1 out]
              "call_1" <- w1027
              "1" <- w1027
            }
            frame 2 {
              w1032 = TRUE
              n649 = Wait (ms)(milliseconds to wait=u32 1000) -> ()  [unwired: 1 out]
              n650 = local write "1"(FALSE) -> ()
              "call_2" <- w1032
              "1 2" <- w1032
            }
            frame 3 {
              w1036 = TRUE
              n651 = local write "1 2"(FALSE) -> ()
              n652 = Wait (ms)(milliseconds to wait=u32 1000) -> ()  [unwired: 1 out]
              "call_3" <- w1036
              "1 3" <- w1036
            }
            frame 4 {
              n653 = Wait (ms)(milliseconds to wait=u32 1000) -> ()  [unwired: 1 out]
              n654 = local write "1 3"(FALSE) -> ()
              "call_back" <- TRUE
            }
            frame 5 {
              n655 = Subtract(x=w1045, y=5 ("x")) -> (x-y=w1044:i32)
              n656 = Wait (ms)(milliseconds to wait=u32 1200 ("millisecond timer value")) -> ()  [unwired: 1 out]
            }
          }
          n657 = feedback-in #39(w1022) -> ()
          n658 = local read "Tab Control"() -> (w1013:enum32{"TAB 1", "TAB 2", "TAB 3", "TAB 4"})
          n659 = Equal?(x=w1013, y=T9."TAB 1" ("Tab Control")) -> (x = y?=w1021:bool)
          n660 = Equal?(x=w1013, y=T9."TAB 6" ("Tab Control")) -> (x = y?=w1015:bool)
          n661 = Equal?(x=w1013, y=T9."TAB 2" ("Tab Control")) -> (x = y?=w1020:bool)
          n662 = Equal?(x=w1013, y=T9."TAB 4" ("Tab Control")) -> (x = y?=w1019:bool)
          n663 = Equal?(x=w1013, y=T9."TAB 7" ("Tab Control")) -> (x = y?=w1014:bool)
          n664 = Equal?(x=w1013, y=T9."TAB 5" ("Tab Control")) -> (x = y?=w1018:bool)
          n665 = Or(x=w1021, y=w1020) -> (x .or. y?=w1017:bool)
          n666 = Or(x=w1015, y=w1014) -> (x .or. y?=w1010:bool)
          n667 = Or(x=w1019, y=w1018) -> (x .or. y?=w1016:bool)
          n668 = Or(x=w1017, y=w1016) -> (x .or. y?=w1012:bool)
          n669 = Or(x=w1012, y=w1010) -> (x .or. y?=w1011:bool)
        }
        n670 = while {
          stop <- w984 stop-if-true
          w983 = FALSE
          n671 = local read "Tab Control"() -> (w994:enum32{"TAB 1", "TAB 2", "TAB 3", "TAB 4"})
          n672 = Equal?(x=w994, y=T9."TAB 1" ("Tab Control")) -> (x = y?=w1002:bool)
          n673 = Equal?(x=w994, y=T9."TAB 2" ("Tab Control")) -> (x = y?=w1001:bool)
          n674 = Equal?(x=w994, y=T9."TAB 4" ("Tab Control")) -> (x = y?=w1000:bool)
          n675 = Equal?(x=w994, y=T9."TAB 5" ("Tab Control")) -> (x = y?=w990:bool)
          n676 = Equal?(x=w994, y=T9."TAB 6" ("Tab Control")) -> (x = y?=w989:bool)
          n677 = Equal?(x=w994, y=T9."TAB 7" ("Tab Control")) -> (x = y?=w986:bool)
          n678 = Or(x=w1002, y=w1001) -> (x .or. y?=w999:bool)
          n679 = Or(x=w1001, y=w1000) -> (x .or. y?=w998:bool)
          n680 = Or(x=w990, y=w989) -> (x .or. y?=w987:bool)
          n681 = Or(x=w999, y=w998) -> (x .or. y?=w988:bool)
          n682 = Or(x=w987, y=w986) -> (x .or. y?=w985:bool)
          n683 = Or(x=w988, y=w985) -> (x .or. y?=w984:bool)
          "Clear 3" <- w984
          n684 = local write "Clear2"(w983) -> ()
          n685 = local write "Clear4"(w983) -> ()
          n686 = local write "Clear1"(w983) -> ()
        }
      }
      frame "TAB 4" {
        n687 = while {
          stop <- w1078 stop-if-true
          n688 = local read "start"() -> (w1070:bool)
          n689 = feedback #40() -> (w1090:i32)  [unwired: 1 in]
          n690 = case shown="True" w1070 {
            tunnel: [w1114 w1115] -> w1091
            tunnel: w1090 -> [w1114 w1116]
            frame False {
            }
            frame True {
              n691 = Increment(x=w1116) -> (x+1=w1115:i32)
            }
          }
          n692 = case shown="4" w1091 {
            selector: w1091 -> [w1093 w1097 w1100 w1105 w1109 w1112]
            tunnel: [w1093 w1097 w1100 w1105 w1109 w1111] -> w1089
            frame 0, Default {
              w1092 = FALSE ("B")
              n693 = local write "ele_back"(w1092) -> ()
              n694 = local write "ele_1"(w1092) -> ()
              n695 = local write "ele_2"(w1092) -> ()
              n696 = local write "ele_3"(w1092) -> ()
            }
            frame 1 {
              w1095 = TRUE
              n697 = local write "BACK_Page4"(FALSE) -> ()
              n698 = Wait (ms)(milliseconds to wait=u32 1500 ("millisecond timer value")) -> ()  [unwired: 1 out]
              "ele_1" <- w1095
              "ele_1" <- w1095
            }
            frame 2 {
              w1099 = TRUE
              n699 = local write "ele_1"(FALSE) -> ()
              n700 = Wait (ms)(milliseconds to wait=u32 1000) -> ()  [unwired: 1 out]
              "ele_2" <- w1099
              "ele_2" <- w1099
            }
            frame 3 {
              w1103 = TRUE
              n701 = local write "ele_2"(FALSE) -> ()
              n702 = Wait (ms)(milliseconds to wait=u32 1000) -> ()  [unwired: 1 out]
              "ele_3" <- w1103
              "ele_3" <- w1103
            }
            frame 4 {
              w1107 = TRUE
              n703 = local write "ele_3"(FALSE) -> ()
              n704 = Wait (ms)(milliseconds to wait=u32 1000) -> ()  [unwired: 1 out]
              "ele_back" <- w1107
              "BACK_Page4" <- w1107
            }
            frame 5 {
              n705 = Subtract(x=w1112, y=5 ("x")) -> (x-y=w1111:i32)
              n706 = Wait (ms)(milliseconds to wait=u32 1200 ("millisecond timer value")) -> ()  [unwired: 1 out]
            }
          }
          n707 = feedback-in #40(w1089) -> ()
          n708 = local read "Tab Control"() -> (w1080:enum32{"TAB 1", "TAB 2", "TAB 3", "TAB 4"})
          n709 = Equal?(x=w1080, y=T9."TAB 1" ("Tab Control")) -> (x = y?=w1088:bool)
          n710 = Equal?(x=w1080, y=T9."TAB 6" ("Tab Control")) -> (x = y?=w1082:bool)
          n711 = Equal?(x=w1080, y=T9."TAB 2" ("Tab Control")) -> (x = y?=w1087:bool)
          n712 = Equal?(x=w1080, y=T9."TAB 3" ("Tab Control")) -> (x = y?=w1086:bool)
          n713 = Equal?(x=w1080, y=T9."TAB 7" ("Tab Control")) -> (x = y?=w1081:bool)
          n714 = Equal?(x=w1080, y=T9."TAB 5" ("Tab Control")) -> (x = y?=w1085:bool)
          n715 = Or(x=w1088, y=w1087) -> (x .or. y?=w1084:bool)
          n716 = Or(x=w1082, y=w1081) -> (x .or. y?=w1077:bool)
          n717 = Or(x=w1086, y=w1085) -> (x .or. y?=w1083:bool)
          n718 = Or(x=w1084, y=w1083) -> (x .or. y?=w1079:bool)
          n719 = Or(x=w1079, y=w1077) -> (x .or. y?=w1078:bool)
        }
        n720 = while {
          stop <- w1051 stop-if-true
          w1050 = FALSE ("Clear1")
          n721 = local read "Tab Control"() -> (w1061:enum32{"TAB 1", "TAB 2", "TAB 3", "TAB 4"})
          n722 = Equal?(x=w1061, y=T9."TAB 1" ("Tab Control")) -> (x = y?=w1069:bool)
          n723 = Equal?(x=w1061, y=T9."TAB 2" ("Tab Control")) -> (x = y?=w1068:bool)
          n724 = Equal?(x=w1061, y=T9."TAB 3" ("Tab Control")) -> (x = y?=w1067:bool)
          n725 = Equal?(x=w1061, y=T9."TAB 5" ("Tab Control")) -> (x = y?=w1057:bool)
          n726 = Equal?(x=w1061, y=T9."TAB 6" ("Tab Control")) -> (x = y?=w1056:bool)
          n727 = Equal?(x=w1061, y=T9."TAB 7" ("Tab Control")) -> (x = y?=w1053:bool)
          n728 = Or(x=w1069, y=w1068) -> (x .or. y?=w1066:bool)
          n729 = Or(x=w1068, y=w1067) -> (x .or. y?=w1065:bool)
          n730 = Or(x=w1057, y=w1056) -> (x .or. y?=w1054:bool)
          n731 = Or(x=w1066, y=w1065) -> (x .or. y?=w1055:bool)
          n732 = Or(x=w1054, y=w1053) -> (x .or. y?=w1052:bool)
          n733 = Or(x=w1055, y=w1052) -> (x .or. y?=w1051:bool)
          "Clear4" <- w1051
          n734 = local write "Clear 3"(w1050) -> ()
          n735 = local write "Clear1"(w1050) -> ()
          n736 = local write "Clear2"(w1050) -> ()
        }
      }
    }
  }
  n737 = while {
    tunnel: w1 -> [w1121]
    tunnel: [w1120] -> w5
    tunnel: w4 -> [w1119]
    tunnel: [w1118] -> w3
    stop <- FALSE stop-if-true
    n738 = case shown="\"TAB 2\"" "Tab Control" {
      selector: "Tab Control" -> [w1131 w1153 w1187 w1196]
      tunnel: [w1130 w1150 w1184 w1194] -> w1117
      frame "TAB 1", Default {
        n739 = local read "Index ที่มากที่สุด"() -> (w1132:i32)
        n740 = local read "ele"() -> (w1129:T1)
        n741 = Add(x=w1131, y=2) -> (x+y=w1125:u32)
        n742 = local read "Index ที่มากที่สุด"() -> (w1136:i32)
        n743 = local read "Index ที่มากที่สุด"() -> (w1135:i32)
        n744 = Equal?(x=w1132, y=0) -> (x = y?=w1146:bool)
        n745 = Increment(x=w1131) -> (x+1=w1140:enum32{"TAB 1", "TAB 2", "TAB 3", "TAB 4"})
        n746 = local read "commu"() -> (w1128:T3)
        n747 = local read "call"() -> (w1134:T2)
        n748 = Add(x=w1125, y=3) -> (x+y=w1124:u32)
        n749 = And(x=w1129, y=w1146) -> (x .and. y?=w1147:T1)
        n750 = Equal?(x=w1136, y=2) -> (x = y?=w1144:bool)
        n751 = Equal?(x=w1135, y=1) -> (x = y?=w1145:bool)
        n752 = And(x=w1134, y=w1145) -> (x .and. y?=w1141:T2)
        n753 = And(x=w1128, y=w1144) -> (x .and. y?=w1142:T3)
        n754 = Select(t=w1124, s=w1147, f=w1131) -> (s? t:f=w1148:u32)
        n755 = Select(t=w1125, s=w1141, f=w1148) -> (s? t:f=w1143:u32)
        n756 = Select(t=w1140, s=w1142, f=w1143) -> (s? t:f=w1130:u32)
        n757 = Wait (ms)(milliseconds to wait=u32 100) -> ()  [unwired: 1 out]
      }
      frame "TAB 2" {
        n758 = local read "Index ที่มากที่สุด"() -> (w1155:i32)
        n759 = local read "Index ที่มากที่สุด"() -> (w1174:i32)
        n760 = local read "Index ที่มากที่สุด"() -> (w1181:i32)
        n761 = local read "Index ที่มากที่สุด"() -> (w1164:i32)
        n762 = local read "ACC"() -> (w1154:T4)
        n763 = local read "Emotion"() -> (w1165:bool)
        n764 = local read "Activity"() -> (w1176:bool)
        n765 = local read "back_page2"() -> (w1182:T5)
        n766 = Equal?(x=w1155, y=2) -> (x = y?=w1157:bool)
        n767 = Equal?(x=w1174, y=0) -> (x = y?=w1175:bool)
        n768 = Decrement(x=w1153) -> (x-1=w1180:enum32{"TAB 1", "TAB 2", "TAB 3", "TAB 4"})
        n769 = Add(x=w1153, y=6) -> (x+y=w1161:u32)
        n770 = Equal?(x=w1164, y=1) -> (x = y?=w1162:bool)
        n771 = Equal?(x=w1181, y=3) -> (x = y?=w1178:bool)
        n772 = Add(x=w1153, y=4) -> (x+y=w1170:u32)
        n773 = Add(x=w1153, y=5) -> (x+y=w1168:u32)
        n774 = And(x=w1154, y=w1157) -> (x .and. y?=w1160:T4)
        n775 = Not(x=w1178) -> (.not. x?=w1177:bool)
        n776 = And(x=w1176, y=w1175) -> (x .and. y?=w1172:bool)
        n777 = And(x=w1165, y=w1162) -> (x .and. y?=w1167:bool)
        n778 = local write "commu"(w1177) -> ()
        n779 = And(x=w1182, y=w1178) -> (x .and. y?=w1179:T5)
        n780 = Select(t=w1161, s=w1160, f=w1153) -> (s? t:f=w1156:u32)
        n781 = Select(t=w1170, s=w1172, f=w1153) -> (s? t:f=w1169:u32)
        n782 = Select(t=w1168, s=w1167, f=w1156) -> (s? t:f=w1152:u32)
        n783 = Select(t=w1180, s=w1179, f=w1169) -> (s? t:f=w1151:u32)
        n784 = Select(t=w1151, s=FALSE, f=w1152) -> (s? t:f=w1150:u32)
      }
      frame "TAB 3" {
        n785 = local read "Index ที่มากที่สุด"() -> (w1192:i32)
        n786 = local read "call_back"() -> (w1189:bool)
        n787 = Subtract(x=w1187, y=2) -> (x-y=w1185:u32)
        n788 = Equal?(x=w1192, y=3) -> (x = y?=w1190:bool)
        n789 = And(x=w1189, y=w1190) -> (x .and. y?=w1191:bool)
        n790 = Not(x=w1190) -> (.not. x?=w1188:bool)
        n791 = local write "call"(w1188) -> ()
        n792 = Select(t=w1185, s=w1191, f=w1187) -> (s? t:f=w1184:u32)
      }
      frame "TAB 4" {
        n793 = local read "Index ที่มากที่สุด"() -> (w1202:i32)
        n794 = local read "BACK_Page4"() -> (w1199:bool)
        n795 = Subtract(x=w1196, y=3) -> (x-y=w1195:u32)
        n796 = Equal?(x=w1202, y=3) -> (x = y?=w1200:bool)
        n797 = And(x=w1199, y=w1200) -> (x .and. y?=w1201:bool)
        n798 = Not(x=w1200) -> (.not. x?=w1198:bool)
        n799 = local write "ele"(w1198) -> ()
        n800 = Select(t=w1195, s=w1201, f=w1196) -> (s? t:f=w1194:u32)
      }
    }
    n801 = local write "Tab Control"(w1117) -> ()
    n802 = Send Notification(notification=w1117, notifier=w1121, error in (no error)=w1119) -> (notifier out=w1120:refnum<notifier>, error out=w1118:errorcluster)
  }
  n803 = Release Notifier(notifier=w5, error in (no error)=w3) -> ()  [unwired: 1 in, 3 out]
  n804 = call <vilib>:"Draw Flattened Pixmap.vi"() -> ()  [unwired: 9 in, 1 out]
  n805 = call <vilib>:"Draw Flattened Pixmap.vi"() -> ()  [unwired: 9 in, 1 out]
  n806 = call <vilib>:"Draw Flattened Pixmap.vi"() -> ()  [unwired: 9 in, 1 out]
